vi "Conus_USB.vi"() -> ()   [LabVIEW 2017]
doc: "Conus USB - Versió bàsica de Conus / Sols adquisició i informe"
uses:
  Instance           2 17Saved   Conus_USB .vi
  Instance           1 17Saved   Conus_USB .vi
  Instance           4 17Saved   Conus_USB .vi
  <vilib>/DAQmx/read.llb/DAQmx Read (Digital 1D Bool NChan 1Samp 1Line).vi
  <vilib>/DAQmx/write.llb/DAQmx Write (Digital 1D Bool NChan 1Samp 1Line).vi
  Control 1.ctl
panel:
  in  "ResetExten":bool caption="TARA"
  in  "Bt_Ini_Exten":bool caption="TARA"
  out "CarregaConfig":bool caption="First time"
  out "IndexCel":u8
  out "Mante_a_Vel_0":bool
  out "Fent_Rep":bool
  out "Booleans":refnum<vi>[](array[refnum])
  in  "Rep. Fetes":u8 caption="N. Rep."
  in  "Salir":bool
  in  "EtiquetaTipusParo":string caption="String"
  in  "Etiqueta Velocitats":string caption="String"
  out "appended array":refnum<vi>[](array[refnum])
  out "MissatgesUsuari":string[](array[string])
  out "Caselles":refnum<vi>[](array[refnum])
  out "StringsEstatMáquina":string[](array[string])
  in  "Rep. A Fer":sgl caption="N. Rep." format="%#_1g"
  out "ParoDefor":bool caption="ParoRotura"
  out "ParoDeforFet":bool caption="ParoProcessat"
  out "ParoCargaFet":bool caption="ParoProcessat"
  out "ParoCarga":bool caption="ParoProcessat"
  in  "CaptadorD":u16(ring) caption="Unidades" items=["Deformación", "Extensómetro"]
  in  "FinalEnsayo":bool caption="Final ensayo"
  in  "ActivaParoCarga":bool caption="ActivaParoDefor"
  in  "ValorParoCarga":sgl caption="Fuerza" min=0 format="%#.3f"
  in  "ActivaParoDefor":bool
  in  "ActivaParoRotura":T1
  in  "ValorParoDesplazamiento":sgl caption="Deformación" min=0 format="%#.3f"
  in  "ValorParoRotura":sgl caption="Rotura (%)" min=0 format="%#_3f"
  out "Ensayo activo":bool caption="Prueba en curso"
  out "ArraiMostresxProva":dbl[](array[numeric])
  out "NMostres":dbl
  in  "BtEliminarUltima":bool=TRUE caption="Eliminar última prueba"
  out "Estado ensayo:":string
  out "CodiAturada":u32
  out "ViuMotor":bool
  out "MotorBipolar":bool
  out "Baixar":bool
  out "Pujar":bool
  out "PrimerCaptador":i32
  out "rings":refnum<vi>[](array[refnum])
  in  "IndexUnitatsD":u8
  in  "IndexUnitatsF":u8
  in  "IndexCaptadorD":u8
  in  "IndexCaptadorF":u8
  out "EtiquetesRegistre":string[](array[string])
  out "start":bool
  out "Active_motor":bool
  in  "Inici x Boto":bool
  out "ExtenPoten":bool caption="Extensòmetre Pot."
  out "ValorSenseTara":dbl
  in  "VelocitatMàxima":dbl
  in  "PerCentPrecarga":sgl=0.5 caption="Precarga (%)"
  in  "Precarga":bool
  in  "BtMaxF":bool
  in  "CaptadorF":u16(ring) caption="Unidades" items=["100 kg"=7, "No presente"=24]
  in  "UnidadesF":u16(ring) caption="Unidades" items=["kg"=0, "N"=1, "daN"=3, "KN"=5]
  in  "BtTaraF":bool caption="TARA"
  out "Fuerza":sgl format="%.2f"
  out "Nº Tests":u8 caption="Tests:"
  out "Sobrecarga":bool
  out "Paro Manual":bool
  out "FCI":bool
  out "FCS":bool
  in  "ResoExten":i8(ring) caption="Resolució Extensometre" items=["0.1", "0.2", "0.5", "0.01", "0.02", "0.05", "0.001", "0.002", "0.005"]
  out "PrecargaOn":bool
  in  "ValorPrecarga":dbl caption="Precarga (%)"
  out "Calibratge D":dbl[](array[numeric])
  out "Extensometre":bool
  in  "UnidadesD":u16(ring) caption="Unidades" items=["mm", "inch"]
  in  "BtTaraD":bool caption="TARA"
  out "Deformacion":sgl caption="Deformación" format="%.1f"
  out "Celula_0":u8
  in  "Células":u8(ring) caption="Célula 1" items=["0.5 kg", "1 Kg", "2 Kg", "5 kg", "10 kg", "20 kg", "50 kg", "100 kg", "200 kg", "300 kg", "500 kg", "1000 kg", "2000 kg", "5000 kg", "10000 kg", "20000 kg", "30000 kg", "P-20 kg", "P-200 kg", "P-500 kg", "P-5000 kg", "P-20000 kg", "P-50 bar", "50000 kg", "No presente"]
  in  "UnidadesF_C2":u16(ring) caption="Unidades" items=["kg"=0, "N"=1, "daN"=3]
  in  "UnidadesF_C1":u16(ring) caption="Unidades" items=["kg"=0, "N"=1, "daN"=3, "KN"=5]
  out "ArraiUnitats":cluster{"String":string, "Value":u16}[](array[cluster])=[{"String"="kg", "Value"=0}, {"String"="N", "Value"=1}, {"String"="g", "Value"=2}, {"String"="daN", "Value"=3}, {"String"="cN", "Value"=4}, {"String"="KN", "Value"=5}, {"String"="lb", "Value"=6}]
  in  "UnitatsF":u8[](array[numeric])
  in  "Velocidad Retorno":sgl caption="Retorno" min=0 max=500 step=1 format="%#.1f"
  in  "Velocidad Ensayo":sgl caption="Ensayo" min=0 max=500 step=1
  out "ValorSobrecargaC2":dbl
  out "Valor de control sobrecarga":dbl
  out "Calibratge":dbl[](array[numeric])
  in  "ParaAssaig":bool
  out "ParoProcessat":bool
  out "Salidas_mando":T2={"HI_down"=TRUE, " LO_down"=TRUE, "HI_up"=TRUE, "*"=TRUE, " LO_up"=TRUE, " start"=TRUE, " Ensayo_down"=TRUE, " Ensayo_up"=TRUE}
  out "VelocitatMotor":dbl min=0.0 max=500.0 step=1.0
  out "TempsLectura":u32=150
  out "Maxim":sgl
  in  "Inhibicio":bool
  in  "Ensayonuevo":bool caption="Ensayo Nuevo"
  in  "Guardar":bool caption="Informe"
  in  "Iniciar / Finalizar":bool=TRUE caption="Finalizar prueba"
  out "TablaFinal":dbl[][](array[numeric])
  out "Tabla":dbl[][](array[numeric])
  in  "Columna":i32
  out "Paro Emergencia":bool
  out "ParoRotura":bool
  out "AssaigMM":bool
  out "DSenseTara":sgl caption="Fuerza - N"
  out "FactorsUnitatsPendents_D":dbl[](array[numeric])
  out "ConversioUnitatsD":dbl[](array[numeric])=[1.0, 9.8756, 1000.0, 0.98]
  in  "DadesAdquirides":dbl[](array[numeric]) format="%#_8g"
  out "FactorsUnitatsPendents_F":dbl[](array[numeric])
  in  "LedAssaig":bool
  out "BaixarMM":bool
  out "PujarMM":bool
  in  "TaraD":sgl
  in  "ValMax":bool
  out "FSenseTara":sgl caption="Fuerza - N"
  in  "TaraF":sgl
  out "Password":string
  out "ValorSobrecargaC1":dbl
  out "ConversioUnitatsF":dbl[](array[numeric])=[1.0, 9.8756, 2.2]
  out "Pendents":dbl[](array[numeric]) format="%#_8g"
  in  "Procesa datos":bool
  in  "Stop":bool=TRUE
  in  "First time":bool
  out "?":cluster{"Y":dbl[], "Y":dbl[]}[](graph)
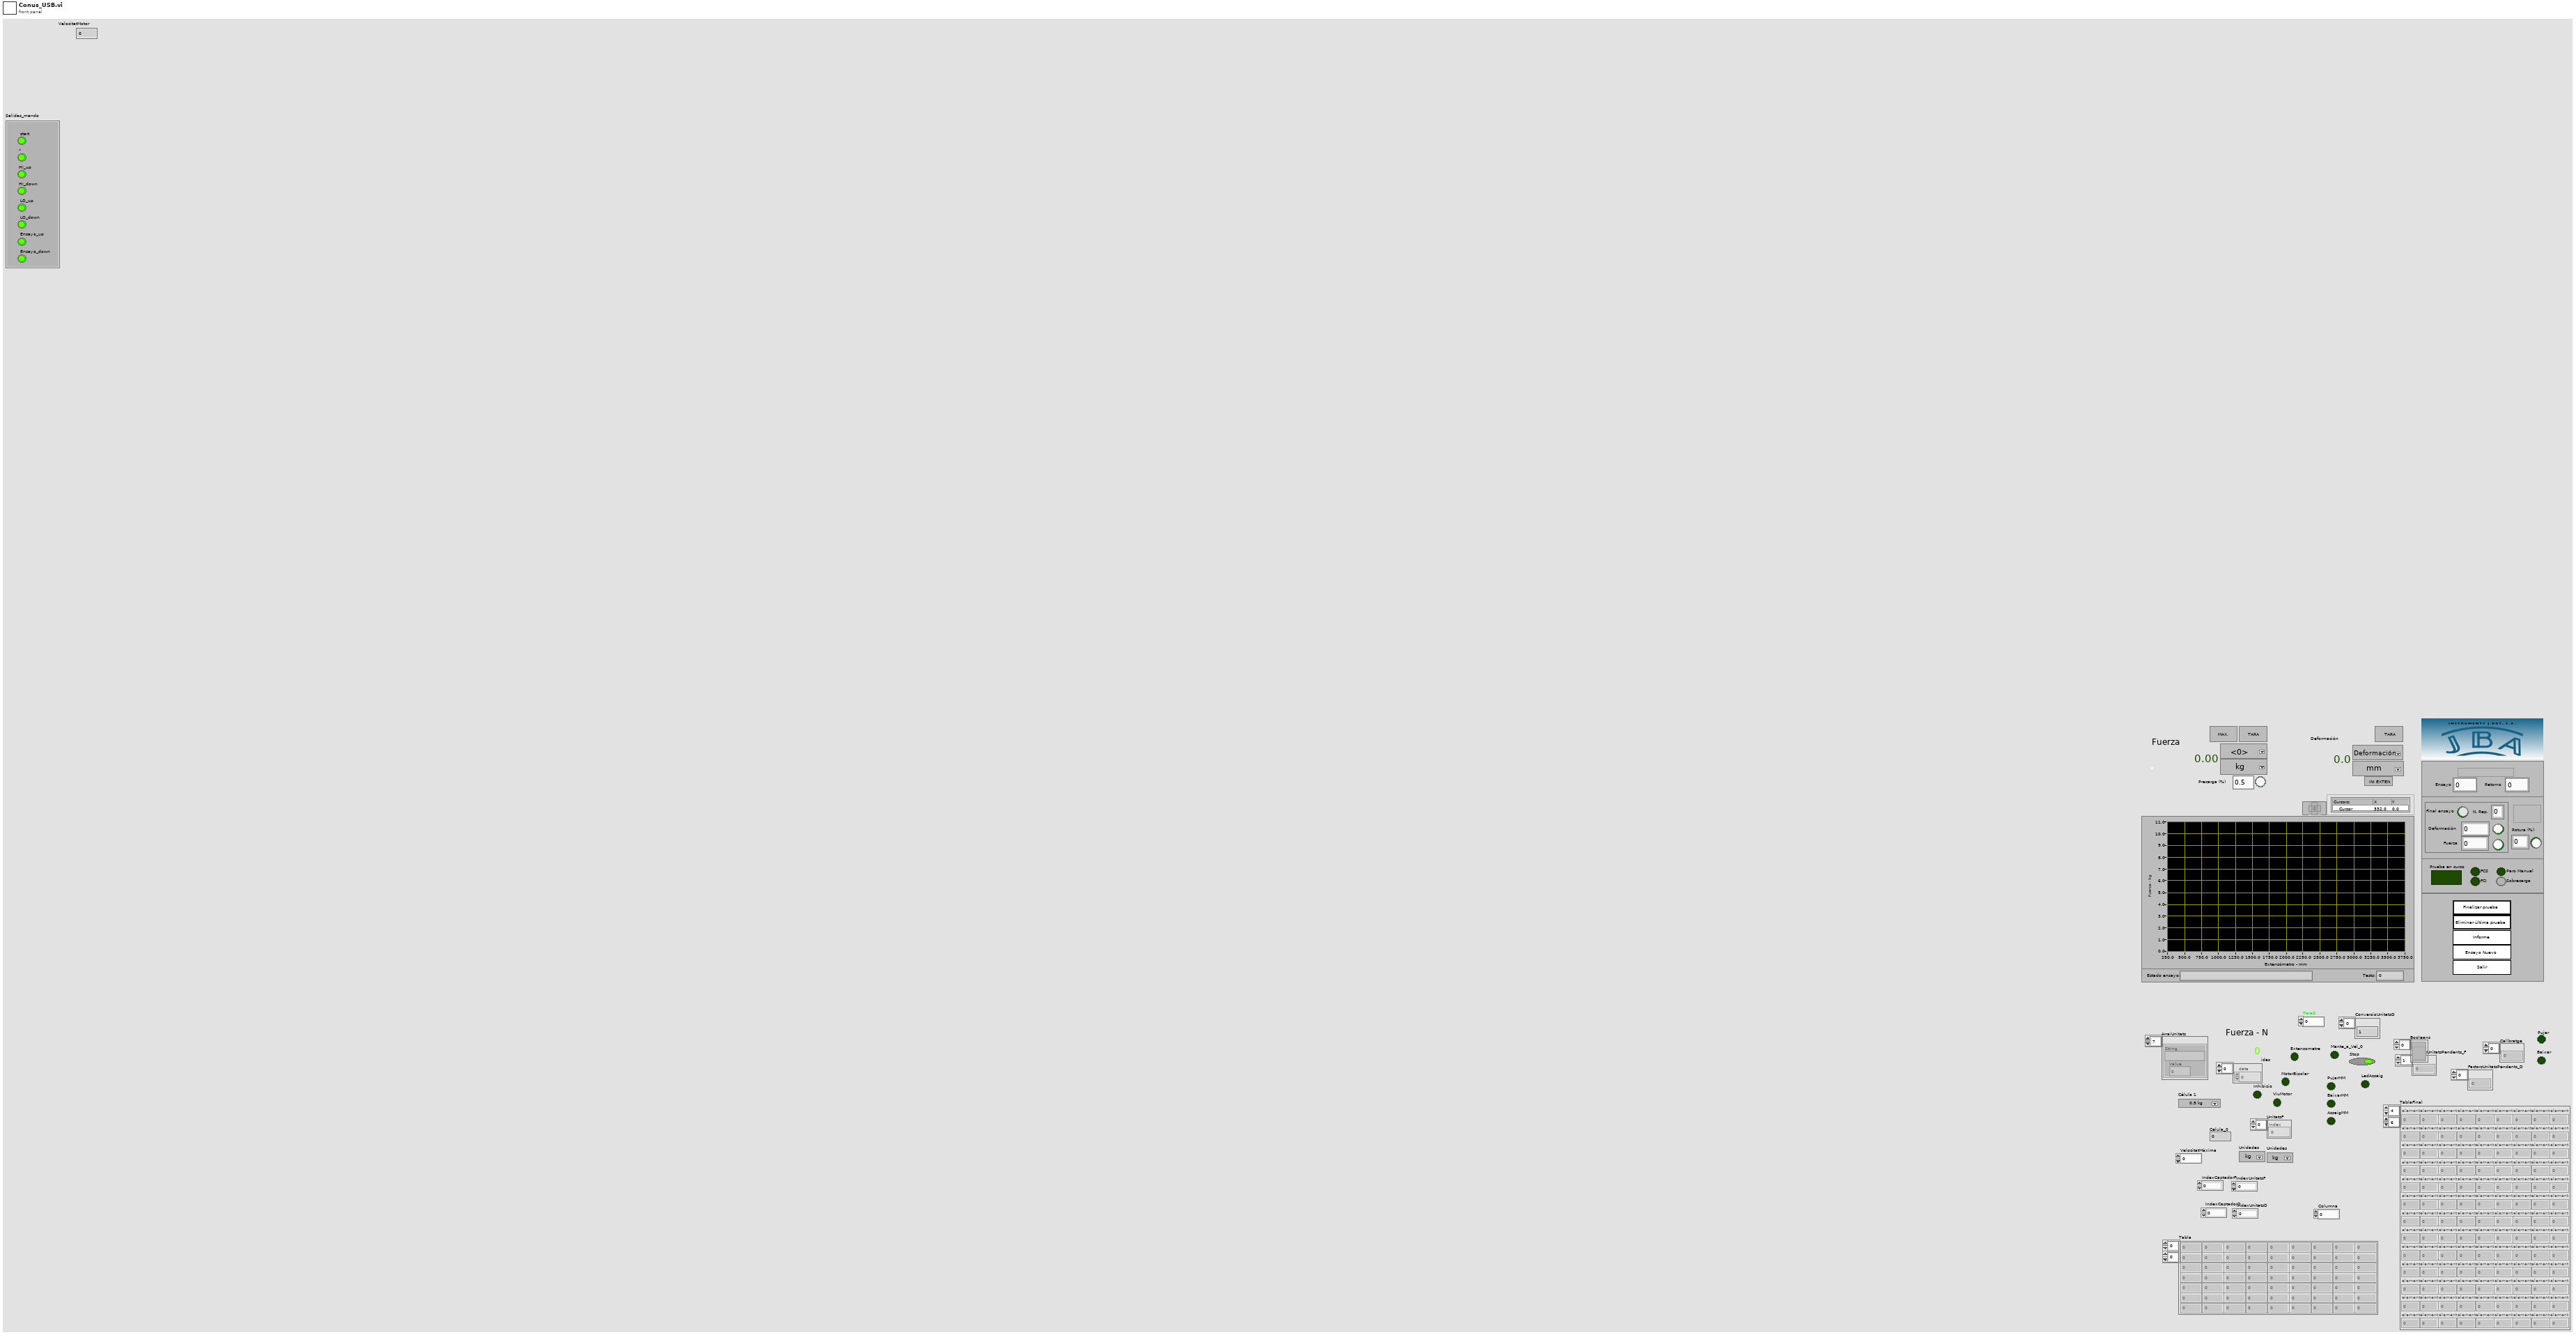
[diagram p1: front panel]
types:
  T1 = typedef "Control 1.ctl" = bool
  T2 = cluster{"HI_down":bool, " LO_down":bool, "HI_up":bool, "*":bool, " LO_up":bool, " start":bool, " Ensayo_down":bool, " Ensayo_up":bool}
  T3 = cluster{"HI_down":bool, "LO_down":bool, "HI_up":bool, "*":bool, "LO_up":bool, "start":bool, "Ensayo_down":bool, "Ensayo_up":bool}
  T4 = typedef "LVStringsAndValuesArrayTypeDef_U8.ctl" = cluster{"String":string, "Value":u8}[]
  T5 = cluster{"Boolean":bool, "element":bool, "Boolean":bool, "Boolean":bool}
  T6 = enum16{"Left Button", "Center Button", "Right Button", "Window Close"}
  T7 = typedef "LVStringsAndValuesArrayTypeDef_U16.ctl" = cluster{"String":string, "Value":u16}[]
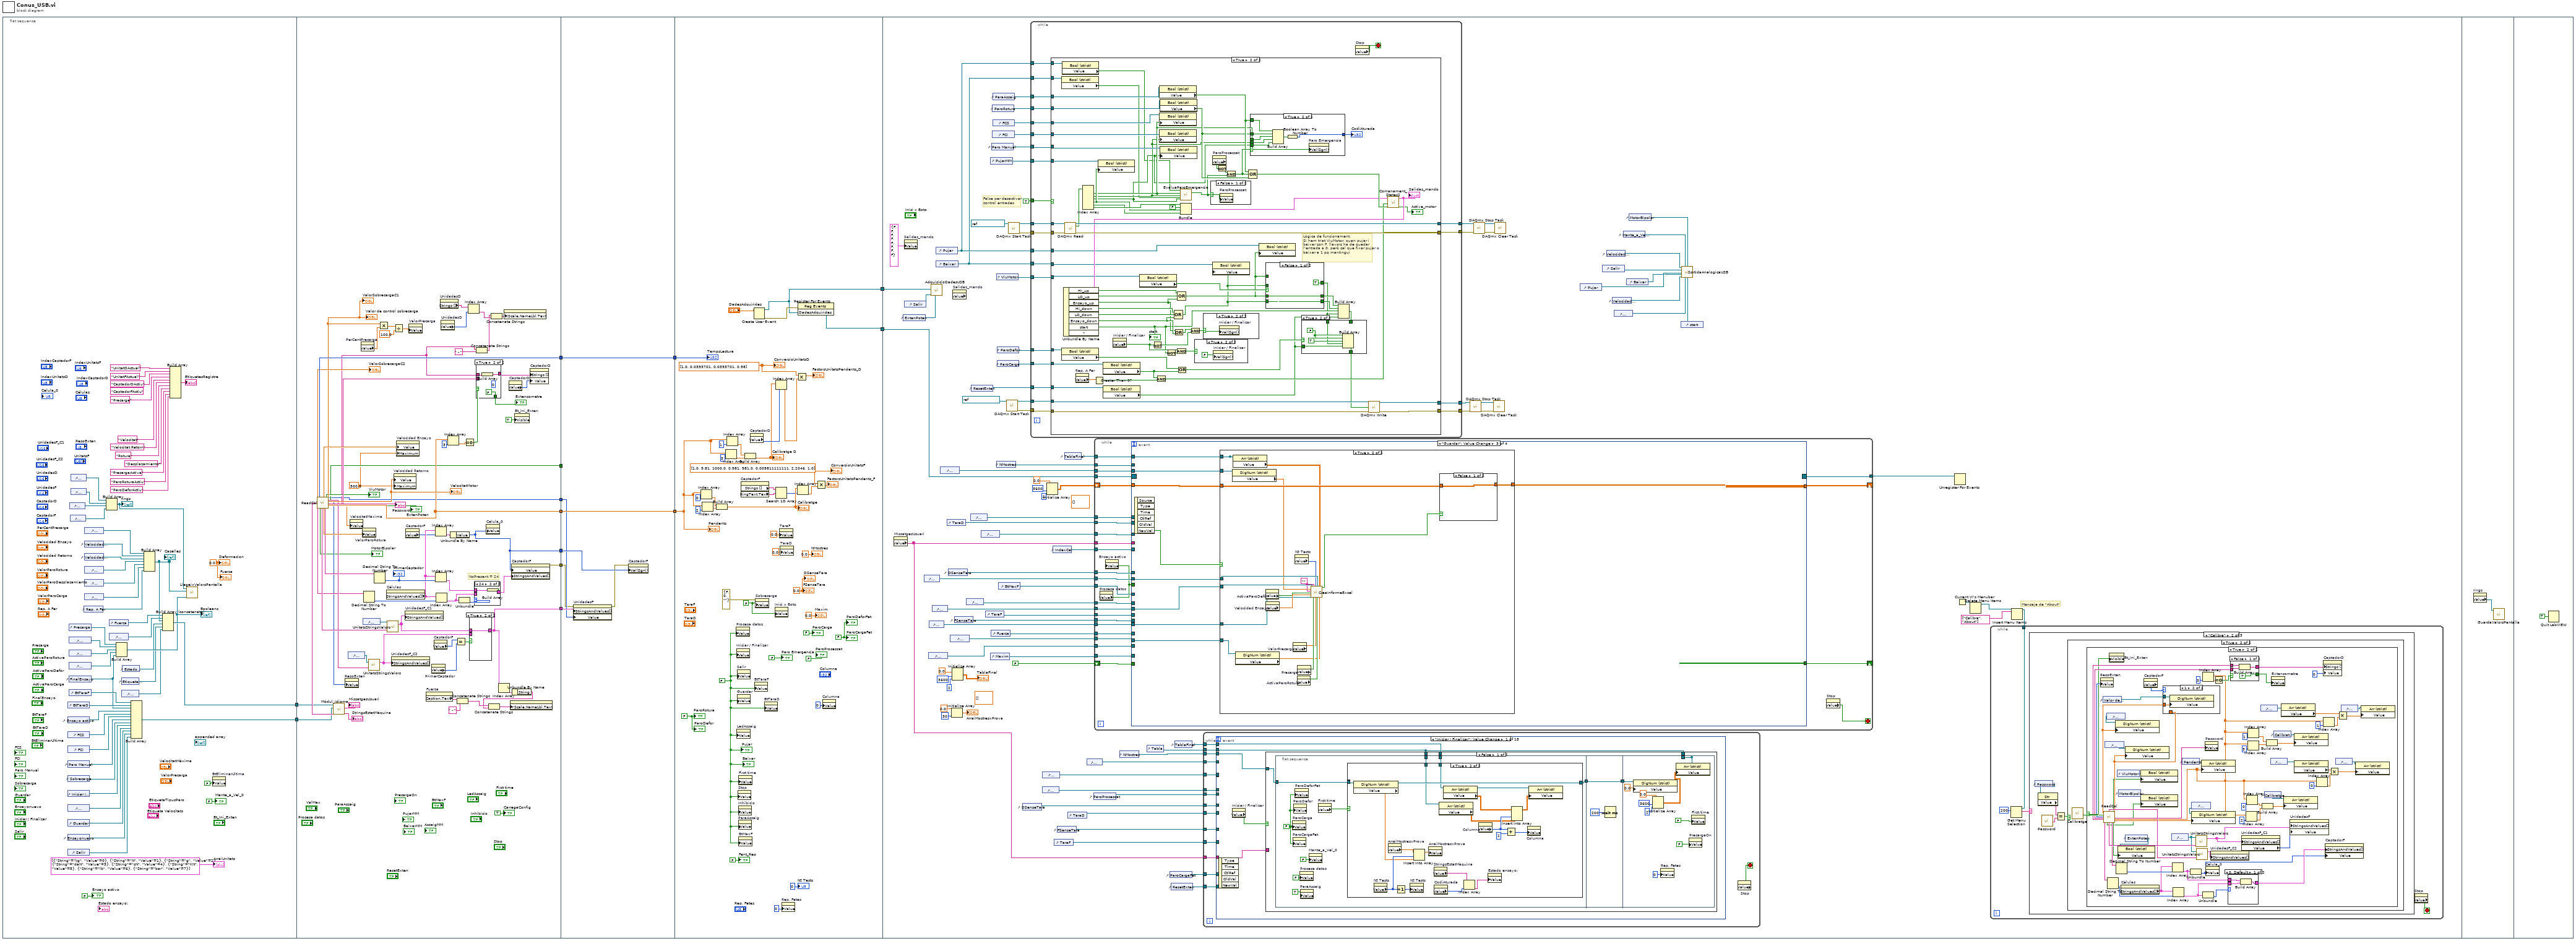
[diagram p0: block diagram]
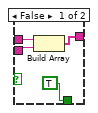
[diagram p3: hidden frame]
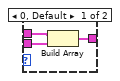
[diagram p4: hidden frame]
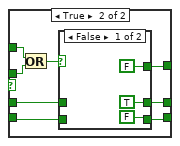
[diagram p7: hidden frame]
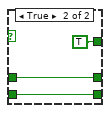
[diagram p8: hidden frame]
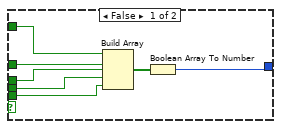
[diagram p11: hidden frame]
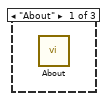
[diagram p13: hidden frame]
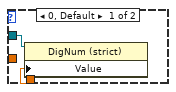
[diagram p16: hidden frame]
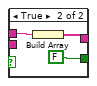
[diagram p17: hidden frame]
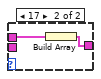
[diagram p18: hidden frame]
diagram:
  n1 = flat-sequence {
    tunnel: [w68] -> w7
    tunnel: [w67] -> w6
    tunnel: [w121] -> w13
    tunnel: [w136] -> w12
    tunnel: w7 -> [w79]
    tunnel: w6 -> [w81]
    tunnel: [w78] -> w5
    tunnel: [w77] -> w4
    tunnel: [w76] -> w3
    tunnel: [w75] -> w2
    tunnel: [w74] -> w1
    tunnel: w13 -> [w159]
    tunnel: [w159] -> w11
    tunnel: w12 -> [w158]
    tunnel: [w158] -> w10
    tunnel: w5 -> [_]
    tunnel: w4 -> [w154]
    tunnel: w3 -> [w157]
    tunnel: w2 -> [w156]
    tunnel: w1 -> [w155]
    tunnel: w11 -> [w178]
    tunnel: [w197] -> w9
    tunnel: [w189] -> w8
    tunnel: w10 -> [w188]
    tunnel: w9 -> [w287]
    tunnel: w8 -> [w270]
    frame #0 {
      w17 = sgl 0.0 ("Deformacion")
      (unwired) "CaptadorFActiu" ("value")
      n2 = control-ref of="BtTaraD"() -> (w42:refnum<vi>)
      n3 = control-ref of="Ensayo activo"() -> (w40:refnum<vi>)
      n4 = control-ref of="FCS"() -> (w39:refnum<vi>)
      n5 = control-ref of="FCI"() -> (w38:refnum<vi>)
      n6 = control-ref of="Paro Manual"() -> (w37:refnum<vi>)
      n7 = control-ref of="Sobrecarga"() -> (w36:refnum<vi>)
      n8 = control-ref of="Iniciar / Finalizar"() -> (w35:refnum<vi>)
      n9 = control-ref of="BtEliminarUltima"() -> (w34:refnum<vi>)
      n10 = control-ref of="Guardar"() -> (w22:refnum<vi>)
      n11 = control-ref of="Ensayonuevo"() -> (w33:refnum<vi>)
      n12 = control-ref of="Salir"() -> (w32:refnum<vi>)
      n13 = control-ref of="Precarga"() -> (w53:refnum<vi>)
      n14 = control-ref of="ActivaParoRotura"() -> (w52:refnum<vi>)
      n15 = control-ref of="ActivaParoDefor"() -> (w51:refnum<vi>)
      n16 = control-ref of="ActivaParoCarga"() -> (w45:refnum<vi>)
      n17 = control-ref of="FinalEnsayo"() -> (w41:refnum<vi>)
      n18 = control-ref of="BtTaraF"() -> (w43:refnum<vi>)
      n19 = control-ref of="CaptadorD"() -> (w48:refnum<vi>)
      n20 = control-ref of="CaptadorF"() -> (w47:refnum<vi>)
      n21 = control-ref of="UnidadesD"() -> (w50:refnum<vi>)
      n22 = control-ref of="UnidadesF"() -> (w49:refnum<vi>)
      n23 = control-ref of="Rep. A Fer"() -> (w15:refnum<vi>)
      n24 = control-ref of="PerCentPrecarga"() -> (w30:refnum<vi>)
      n25 = control-ref of="Velocidad Ensayo"() -> (w29:refnum<vi>)
      n26 = control-ref of="Velocidad Retorno"() -> (w54:refnum<vi>)
      n27 = control-ref of="ValorParoRotura"() -> (w28:refnum<vi>)
      n28 = control-ref of="ValorParoDesplazamiento"() -> (w27:refnum<vi>)
      n29 = control-ref of="ValorParoCarga"() -> (w26:refnum<vi>)
      n30 = Build Array(w50, w49, w48, w47) -> (w46:refnum<vi>[])
      "rings" <- w46
      n31 = control-ref of="Fuerza"() -> (w25:refnum<vi>)
      n32 = control-ref of="Deformacion"() -> (w24:refnum<vi>)
      n33 = Build Array(w53, w52, w51, w45, w41) -> (w31:refnum<vi>[])
      "Booleans" <- w31
      n34 = control-ref of="Etiqueta Velocitats"() -> (w19:refnum<vi>)
      n35 = control-ref of="EtiquetaTipusParo"() -> (w18:refnum<vi>)
      n36 = control-ref of="Estado ensayo:"() -> (w20:refnum<vi>)
      n37 = Build Array(w43, w42, w41, w40, w39, w38, w37, w36, w35, w34, w22, w33, w32) -> (w68:refnum<vi>[])
      n38 = Build Array(w30, w29, w54, w28, w27, w26, w15) -> (w21:refnum<vi>[])
      "Caselles" <- w21
      n39 = Build Array (concatenate)(w25, w24, w21, w20, w19, w18) -> (w67:refnum<vi>[])
      n40 = Build Array("UnitatDActual" ("value"), "UnitatFActual" ("value"), "CaptadorDActiu" ("value"), "Precarga" ("value"), "Velocitat" ("value"), "Velocitat Retorn" ("value"), "Rotura" ("value"), "Desplazamiento" ("value"), "PrecargaActiva" ("value"), "ParoRoturaActiu" ("value"), "ParoDeforActiu" ("value")) -> (→"EtiquetesRegistre":string[])
      n41 = call "LlegeixValorsPantalla.vi"("rings"=w46, "Caselles 2"=w21, "Booleans"=w31) -> ()  [unwired: 8 in]
      n42 = property on="BtEliminarUltima" class="Bool (strict)"("Value"=FALSE ("BtEliminarUltima")) -> ()  [unwired: 2 in, 2 out]
      "Ensayo activo" <- FALSE ("Ensayo activo")
      "Fuerza" <- w17
      "Deformacion" <- w17
      "ArraiUnitats" <- cluster{"String":string, "Value":u16}[] [{"String"="kg", "Value"=0}, {"String"="N", "Value"=1}, {"String"="g", "Value"=2}, {"String"="daN", "Value"=3}, {"String"="cN", "Value"=4}, {"String"="KN", "Value"=5}, {"String"="lb", "Value"=6}, {"String"="bar", "Value"=7}] ("Strings And Values [] 2")
      "Mante_a_Vel_0" <- FALSE ("Mante_a_Vel_0")
    }
    frame #1 {
      w71 = 500.0 ("Data Entry Limits:Maximum")
      # "NoPresent = 24"
      n43 = call "ReadCal.vi"() -> ("SobrecargaC2"=→"ValorSobrecargaC2":dbl, "ResoExten"=w114:i8, "TextExtensometre"=w118:string, "TextDeformacio"=w80:string, "SegonCaptador"=w128:string, "TempsLectura"=w136:u16, "Idioma"=w83:string, "MotorBipolar"=→"MotorBipolar":bool, "UnitatsC2"=w129:string, "UnitatsC1"=w130:string, "Velocitat"=w137:dbl, "ParoRotura"=w138:dbl, "V. Retorn"=w133:dbl, "PrimerCaptador"=w126:string, "ViuMotor"=→"ViuMotor":bool, "ExtenPoten"=→"ExtenPoten":bool, "Unidades"=w74:u8, "Sec?"=w78:bool, "SobrecargaC1"=w115:dbl, "Password"=→"Password":string, "Pendents"=w121:dbl[], "VelocitatMàxima"=w70:dbl)  [unwired: 2 in, 4 out]
      "VelocitatMotor" <- w133
      "ValorSobrecargaC1" <- w115
      "Valor de control sobrecarga" <- w115
      n44 = call "Módul_Idioma.vi"("Idioma"=w83, "Array"=w79, "Caselles"=w81) -> ("TextosEstatMaquina"=→"StringsEstatMáquina":string[], "MissatgesUsuari"=→"MissatgesUsuari":string[])  [unwired: 7 in]
      n45 = property on="ResoExten" class="Ring (strict)"("Value"=w114) -> ()  [unwired: 2 in, 2 out]
      n46 = control-ref of="ArraiUnitats"() -> (w131:refnum<vi>)
      n47 = property on="VelocitatMàxima" class="DigNum (strict)"("Value"=w70) -> ()  [unwired: 2 in, 2 out]
      n48 = property on="PerCentPrecarga" class="DigNum (strict)"() -> ("Value"=w106:sgl)  [unwired: 2 in, 2 out]
      n49 = property on="ValorParoRotura" class="DigNum (strict)"("Value"=w138) -> ()  [unwired: 2 in, 2 out]
      n50 = control-ref of="ArraiUnitats"() -> (w132:refnum<vi>)
      n51 = Decimal String To Number(string=w128) -> (number=w127:i32)  [unwired: 2 in, 1 out]
      n52 = call "UnitatsStringsValors.vi"("UnitatsC1"=w129, "Arr Refnum"=w131) -> ("Array 2"=w96:cluster{"String":string, "Value":u16}[])  [unwired: 1 out]
      n53 = Decimal String To Number(string=w126) -> (number=w125:i32)  [unwired: 2 in, 1 out]
      "PrimerCaptador" <- w125
      n54 = Multiply(x=w115, y=w106) -> (x*y=w117:dbl)
      n55 = property on="Células" class="Ring (strict)"() -> ("StringsAndValues[]"=w103:T4)  [unwired: 2 in, 2 out]
      n56 = call "UnitatsStringsValors.vi"("UnitatsC1"=w130, "Arr Refnum"=w132) -> ("Array 2"=w97:cluster{"String":string, "Value":u16}[])  [unwired: 1 out]
      n57 = property on="UnidadesF_C2" class="Ring (strict)"("StringsAndValues[]"=w96) -> ()  [unwired: 2 in, 2 out]
      n58 = Divide(x=w117, y=100.0) -> (x/y=w112:dbl)
      n59 = property on="Velocidad Retorno" class="DigNum (strict)"("Value"=w133, "Maximum"=w71) -> ()  [unwired: 2 in, 2 out]
      n60 = property on="Velocidad Ensayo" class="DigNum (strict)"("Value"=w137, "Maximum"=w71) -> ()  [unwired: 2 in, 2 out]
      n61 = property on="UnidadesF_C1" class="Ring (strict)"("StringsAndValues[]"=w97) -> ()  [unwired: 2 in, 2 out]
      n62 = property on="CaptadorF" class="Ring (strict)"() -> ("Value"=w101:u16)  [unwired: 2 in, 2 out]
      n63 = property on="ValorPrecarga" class="DigNum (strict)"("Value"=w112) -> ()  [unwired: 2 in, 2 out]
      n64 = property on="Fuerza" class="DigNum (strict)"() -> ("Caption.Text"=w109:string)  [unwired: 2 in, 2 out]
      n65 = property on="PrimerCaptador" class="DigNum (strict)"() -> ("Value"=w98:i32)  [unwired: 2 in, 2 out]
      n66 = property on="CaptadorF" class="Ring (strict)"() -> ("Value"=w99:u16)  [unwired: 2 in, 2 out]
      n67 = Index Array(array=w103, index=w101) -> (element=w102:cluster{"String":string, "Value":u8})
      n68 = Index Array(array=w103, index=w125) -> (element=w105:cluster{"String":string, "Value":u8})
      n69 = Index Array(array=w103, index=w127) -> (element=w123:cluster{"String":string, "Value":u8})
      n70 = property on="UnidadesD" class="Ring (strict)"() -> ("Strings []"=w91:string[])  [unwired: 2 in, 2 out]
      n71 = property on="UnidadesD" class="Ring (strict)"() -> ("Value"=w90:u16)  [unwired: 2 in, 2 out]
      n72 = Index Array(array=w121, index=3) -> (element=w119:dbl)
      n73 = Unbundle By Name(w102) -> ("Value"=w76:u8)
      n74 = Equal?(x=w99, y=w98) -> (x = y?=w100:bool)
      n75 = Concatenate Strings(w109, " - ") -> (w108:string)
      n76 = Unbundle(w123) -> ("Value"=w124:u8)  [unwired: 1 out]
      n77 = Equal To 0?(x=w119) -> (x = 0?=w122:bool)
      n78 = Index Array(array=w91, index=w90) -> (element=w89:string)
      n79 = case shown="True" w100 {
        tunnel: w97 -> [_ w140]
        tunnel: [w139 w140] -> w75
        tunnel: w96 -> [w139 _]
        frame False {
        }
        frame True {
        }
      }
      n80 = case shown="24" w124 {
        tunnel: w105 -> [w150 w151]
        tunnel: w123 -> [w149 _]
        tunnel: [w148 w152] -> w104
        frame 0, Default {
          n81 = Build Array(w150, w149) -> (w148:cluster{"String":string, "Value":u8}[])
        }
        frame 24 {
          n82 = Build Array(w151) -> (w152:cluster{"String":string, "Value":u8}[])
        }
      }
      n83 = Concatenate Strings(w80, " - ") -> (w87:string)
      n84 = case shown="True" w122 {
        tunnel: w118 -> [w144 _]
        tunnel: [w143 w145] -> w92
        tunnel: [TRUE ("Extensometre") FALSE ("Extensometre")] -> w72
        tunnel: w80 -> [w141 w146]
        frame False {
          n85 = Build Array(w141, w144) -> (w143:string[])
        }
        frame True {
          (unwired) 0 ("index")
          n86 = Build Array(w146) -> (w145:string[])
        }
      }
      "Extensometre" <- w72
      n87 = property on="Celula_0" class="DigNum (strict)"("Value"=w76) -> ()  [unwired: 2 in, 2 out]
      n88 = Concatenate Strings(w87, w89) -> (w107:string)
      n89 = Index Array(array=w75) -> (element=w94:cluster{"String":string, "Value":u16})  [unwired: 1 in]
      n90 = property class="XYGraph (strict)"("XScale.NameLbl.Text"=w107) -> ()  [unwired: 2 in, 2 out]
      n91 = property on="CaptadorD" class="Ring (strict)"() -> ("Value"=w93:u16)  [unwired: 2 in, 2 out]
      n92 = property on="CaptadorF" class="Ring (strict)"("Value"=w76, "StringsAndValues[]"=w104) -> (error out=w77:errorcluster)  [unwired: 2 in, 1 out]
      n93 = Unbundle By Name(w94) -> ("String"=w95:string)
      n94 = Concatenate Strings(w108, w95) -> (w113:string)
      n95 = property class="XYGraph (strict)"("YScale.NameLbl.Text"=w113) -> ()  [unwired: 2 in, 2 out]
      n96 = property on="Bt_Ini_Exten" class="Bool (strict)"("Visible"=TRUE) -> ()  [unwired: 2 in, 2 out]
      n97 = property on="CaptadorD" class="Ring (strict)"("Strings []"=w92, "Value"=w93) -> ()  [unwired: 2 in, 2 out]
      "CarregaConfig" <- TRUE ("CarregaConfig")
    }
    frame #2 {
      n98 = property on="UnidadesF" class="Ring (strict)"(error in=w154, "StringsAndValues[]"=w156, "Value"=w155) -> (error out=w153:errorcluster)  [unwired: 1 in, 1 out]
      n99 = property on="CaptadorF" class="Ring (strict)"(error in=w153, "Val(Sgnl)"=w157) -> ()  [unwired: 1 in, 2 out]
    }
    frame #3 {
      w163 = FALSE ("ParoCargaFet")
      w162 = FALSE ("ParoRotura")
      w176 = dbl[] [1.0, 0.0393701, 0.0393701, 0.98]
      w191 = sgl 0.0 ("FSenseTara")
      w199 = dbl[] [1.0, 9.81, 1000.0, 0.981, 981.0, 0.009811111111, 2.2046, 1.0]
      w170 = FALSE ("Sobrecarga")
      w166 = FALSE ("Iniciar / Finalizar")
      n100 = Index Array(array=w178, index=0) -> (element=w184:dbl)
      n101 = Index Array(array=w178, index=2) -> (element=w185:dbl)
      n102 = Build Array(w184, w185) -> (w183:dbl[])
      "Calibratge" <- w183
      n103 = Index Array(array=w178, index=3) -> (element=w179:dbl)
      n104 = Index Array(array=w178, index=1) -> (element=w177:dbl)
      n105 = property on="Procesa datos" class="Bool (strict)"("Value"=w166) -> ()  [unwired: 2 in, 2 out]
      n106 = property on="Iniciar / Finalizar" class="Bool (strict)"("Value"=w166) -> ()  [unwired: 2 in, 2 out]
      n107 = property on="LedAssaig" class="Bool (strict)"("Value"=w166) -> ()  [unwired: 2 in, 2 out]
      n108 = property on="Salir" class="Bool (strict)"("Value"=w166) -> ()  [unwired: 2 in, 2 out]
      n109 = property on="Guardar" class="Bool (strict)"("Value"=w166) -> ()  [unwired: 2 in, 2 out]
      n110 = property on="Stop" class="Bool (strict)"("Value"=w166) -> ()  [unwired: 2 in, 2 out]
      n111 = property on="Inhibicio" class="Bool (strict)"("Value"=w166) -> ()  [unwired: 2 in, 2 out]
      n112 = property on="ParaAssaig" class="Bool (strict)"("Value"=w166) -> ()  [unwired: 2 in, 2 out]
      n113 = property on="First time" class="Bool (strict)"("Value"=w166) -> ()  [unwired: 2 in, 2 out]
      n114 = property on="BtMaxF" class="Bool (strict)"("Value"=w166) -> ()  [unwired: 2 in, 2 out]
      n115 = property on="CaptadorF" class="Ring (strict)"() -> ("Strings []"=w169:string[], "RingText.Text"=w168:string)  [unwired: 2 in, 2 out]
      n116 = Build Array(w177, w179) -> (w174:dbl[])
      "Calibratge D" <- w174
      n117 = property on="CaptadorD" class="Ring (strict)"() -> ("Value"=w175:u16)  [unwired: 2 in, 2 out]
      n118 = Create User Event(user event datatype="DadesAdquirides") -> (user event=w189:refnum<user-event>, error out=w196:errorcluster)  [unwired: 1 in]
      n119 = property on="BtTaraF" class="Bool (strict)"("Value"=w166) -> ()  [unwired: 2 in, 2 out]
      n120 = property on="Sobrecarga" class="Bool (strict)"(error in=errorcluster {"status"=FALSE, "code"=0, "source"=""} ("error in (no error)"), "Value"=w170) -> ()  [unwired: 1 in, 2 out]
      n121 = property on="BtTaraD" class="Bool (strict)"("Value"=w166) -> ()  [unwired: 2 in, 2 out]
      n122 = property on="Inici x Boto" class="Bool (strict)"("Value"=w170) -> ()  [unwired: 2 in, 2 out]
      n123 = Index Array(array=w174, index=w175) -> (element=w173:dbl)
      n124 = Search 1D Array(1D array=w169, element=w168) -> (index of element=w167:i32)  [unwired: 1 in]
      n125 = property on="TaraF" class="DigNum (strict)"("Value"=sgl 0.0 ("Tara")) -> ()  [unwired: 2 in, 2 out]
      n126 = property on="TaraD" class="DigNum (strict)"("Value"=sgl 0.0 ("TaraD")) -> ()  [unwired: 2 in, 2 out]
      n127 = property on="Rep. Fetes" class="DigNum (strict)"("Value"=u8 0 ("Rep. Fetes")) -> ()  [unwired: 2 in, 2 out]
      n128 = Multiply(x=w176, y=w173) -> (x*y=→"FactorsUnitatsPendents_D":dbl[])
      n129 = Index Array(array=w183, index=w167) -> (element=w182:dbl)
      n130 = register-events(error in=w196, w189) -> (reference out=w197:refnum<event-registration>)  [unwired: 1 in, 1 out]
      n131 = Multiply(x=w199, y=w182) -> (x*y=→"FactorsUnitatsPendents_F":dbl[])
      n132 = property on="Columna" class="DigNum (strict)"("Value"=0 ("Columna")) -> ()  [unwired: 2 in, 2 out]
      "Pendents" <- w178
      "ConversioUnitatsF" <- w199
      "FSenseTara" <- w191
      "ConversioUnitatsD" <- w176
      "DSenseTara" <- w191
      "ParoRotura" <- w162
      "Paro Emergencia" <- FALSE ("Paro Emergencia")
      "Maxim" <- sgl 0.0 ("Maxim")
      "TempsLectura" <- w188
      "ParoProcessat" <- FALSE ("ParoProcessat")
      "Nº Tests" <- u8 0 ("Nº Tests")
      "Pujar" <- w166
      "Baixar" <- w166
      "NMostres" <- 0.0 ("NMostres")
      "ParoCarga" <- FALSE ("ValorCargaFet")
      "ParoCargaFet" <- w163
      "ParoDeforFet" <- w163
      "ParoDefor" <- w162
      "Fent_Rep" <- FALSE ("Fent_Rep")
    }
    frame #4 {
      (unwired) dbl[][] []
      (unwired) dbl[][] [] ("TablaFinal")
      # "False per desactivar\ncontrol entrades"
      # "Mensaje de \"About\""
      n133 = property on="MissatgesUsuari" class="Arr (strict)"() -> ("Value"=w217:string[])  [unwired: 2 in, 2 out]
      n134 = control-ref of="ExtenPoten"() -> (w237:refnum<vi>)
      n135 = property on="Salidas_mando" class="Clust (strict)"("Value"=T3 {"HI_down"=FALSE, "LO_down"=FALSE, "HI_up"=FALSE, "*"=FALSE, "LO_up"=FALSE, "start"=FALSE, "Ensayo_down"=FALSE, "Ensayo_up"=FALSE} ("Salidas_mando")) -> ()  [unwired: 2 in, 2 out]
      n136 = control-ref of="Salir"() -> (w271:refnum<vi>)
      n137 = control-ref of="UnidadesD"() -> (w280:refnum<vi>)
      n138 = control-ref of="ValorParoCarga"() -> (w222:refnum<vi>)
      n139 = control-ref of="CaptadorF"() -> (w246:refnum<vi>)
      n140 = call "AdquisicioDadesUSB.vi"("ExtensometrePoten"=w237, "Stop"=w271, "user event"=w270) -> ()  [unwired: 9 in]
      n141 = control-ref of="UnidadesF"() -> (w279:refnum<vi>)
      n142 = control-ref of="Pujar"() -> (w228:refnum<vi>)
      n143 = control-ref of="Baixar"() -> (w227:refnum<vi>)
      n144 = control-ref of="ValorParoDesplazamiento"() -> (w242:refnum<vi>)
      n145 = control-ref of="TaraD"() -> (w283:refnum<vi>)
      n146 = control-ref of="DSenseTara"() -> (w284:refnum<vi>)
      n147 = control-ref of="ValorParoRotura"() -> (w276:refnum<vi>)
      n148 = Initialize Array(0.0 ("element"), 30 ("dimension size")) -> (→"ArraiMostresxProva":dbl[])
      n149 = Initialize Array(0.0 ("element"), 3600 ("dimension size"), 2 ("dimension size")) -> (→"TablaFinal":dbl[][])
      n150 = property on="Salidas_mando" class="Clust (strict)" props=["Value"]() -> ()  [unwired: 2 in, 3 out]
      n151 = control-ref of="FSenseTara"() -> (w289:refnum<vi>)
      n152 = control-ref of="FactorsUnitatsPendents_F"() -> (w288:refnum<vi>)
      n153 = control-ref of="FactorsUnitatsPendents_D"() -> (w286:refnum<vi>)
      n154 = control-ref of="ResetExten"() -> (w209:refnum<vi>)
      n155 = control-ref of="Deformacion"() -> (w285:refnum<vi>)
      n156 = control-ref of="TaraF"() -> (w290:refnum<vi>)
      n157 = control-ref of="PujarMM"() -> (w230:refnum<vi>)
      n158 = control-ref of="Maxim"() -> (w269:refnum<vi>)
      n159 = control-ref of="Fuerza"() -> (w239:refnum<vi>)
      n160 = control-ref of="Paro Manual"() -> (w250:refnum<vi>)
      n161 = control-ref of="ParoRotura"() -> (w249:refnum<vi>)
      n162 = control-ref of="FCI"() -> (w251:refnum<vi>)
      n163 = control-ref of="ParaAssaig"() -> (w248:refnum<vi>)
      n164 = control-ref of="FCS"() -> (w252:refnum<vi>)
      n165 = control-ref of="ViuMotor"() -> (w231:refnum<vi>)
      n166 = control-ref of="NMostres"() -> (w223:refnum<vi>)
      n167 = control-ref of="ParoDefor"() -> (w220:refnum<vi>)
      n168 = control-ref of="ParoCarga"() -> (w221:refnum<vi>)
      n169 = control-ref of="BtMaxF"() -> (w244:refnum<vi>)
      n170 = call <vilib>:"DAQmx Start Task.vi"("task/channels in"=refnum<k21> "USBDigitalOut") -> ("task out"=w258:refnum<k21>, "error out"=w257:errorcluster)  [unwired: 13 in]
      n171 = call <vilib>:"DAQmx Start Task.vi"("task/channels in"=refnum<k21> "USBDigitalIn") -> ("task out"=w266:refnum<k21>, "error out"=w265:errorcluster)  [unwired: 13 in]
      n172 = control-ref of="DSenseTara"() -> (w281:refnum<vi>)
      n173 = while {
        tunnel: w266 -> [w317]
        tunnel: w265 -> [w316]
        tunnel: [w315] -> w261
        tunnel: [w314] -> w260
        tunnel: w258 -> [w313]
        tunnel: w257 -> [w312]
        tunnel: [w311] -> w254
        tunnel: [w310] -> w253
        tunnel: w252 -> [w309]
        tunnel: w251 -> [w308]
        tunnel: w250 -> [w307]
        tunnel: w249 -> [w306]
        tunnel: w248 -> [w305]
        tunnel: TRUE -> [w304]
        tunnel: w228 -> [w302]
        tunnel: w227 -> [w301]
        tunnel: w231 -> [w300]
        tunnel: w230 -> [w299]
        tunnel: w227 -> [w298]
        tunnel: w228 -> [w297]
        tunnel: w221 -> [w296]
        tunnel: w220 -> [w295]
        tunnel: w209 -> [w294]
        stop <- w303 stop-if-true
        n174 = case shown="True" w304 {
          tunnel: w317 -> [w321 w392]
          tunnel: w316 -> [w320 w391]
          tunnel: [w321 w390] -> w315
          tunnel: [w320 w389] -> w314
          tunnel: w313 -> [w319 w384]
          tunnel: w312 -> [w318 w383]
          tunnel: [w318 w382] -> w311
          tunnel: [w319 w381] -> w310
          tunnel: w309 -> [_ w378]
          tunnel: w308 -> [_ w377]
          tunnel: w307 -> [_ w376]
          tunnel: w306 -> [_ w369]
          tunnel: w305 -> [_ w366]
          tunnel: w302 -> [_ w359]
          tunnel: w301 -> [_ w358]
          tunnel: w300 -> [_ w356]
          tunnel: w299 -> [_ w346]
          tunnel: w298 -> [_ w343]
          tunnel: w297 -> [_ w342]
          tunnel: w296 -> [_ w333]
          tunnel: w295 -> [_ w332]
          tunnel: w294 -> [_ w324]
          frame False {
          }
          frame True {
            # "Lògica de funcionament.\nSi hem triat ViuMotor, quan pujar i baixar son F, llavors ha de quedar l'entrada a 0, però cal que fixar pujar o baixar a 1 pq mantingui"
            n175 = property class="Bool (strict)"(reference=w343) -> ("Value"=w336:bool)  [unwired: 1 in, 2 out]
            n176 = property class="Bool (strict)"(reference=w332) -> ("Value"=w331:bool)  [unwired: 1 in, 2 out]
            n177 = property class="Bool (strict)"(reference=w342) -> ("Value"=w337:bool)  [unwired: 1 in, 2 out]
            n178 = call-poly <vilib>:"DAQmx Read.vi"("task/channels in"=w392, "error in"=w391) -> ("task out"=w390:refnum<k21>, "data"=w350:bool[], "error out"=w389:errorcluster)  [unwired: 11 in]
            n179 = property on="Rep. A Fer" class="DigNum (strict)"() -> ("Value"=w328:sgl)  [unwired: 2 in, 2 out]
            n180 = Index Array(array=w350) -> (element #1=w340:bool, element #2=w339:bool, element #3=w338:bool, element #4=w344:bool, element #5=w345:bool, element #6=w380:bool)  [unwired: 6 in]
            n181 = Greater Than 0?(x=w328) -> (x > 0?=w326:bool)
            n182 = property class="Bool (strict)"(reference=w346, "Value"=w344) -> ()  [unwired: 1 in, 2 out]
            n183 = property class="Bool (strict)"(reference=w333) -> ("Value"=w327:bool)  [unwired: 1 in, 2 out]
            n184 = property class="Bool (strict)"(reference=w324) -> ("Value"=w322:bool)  [unwired: 1 in, 2 out]
            n185 = property on="Iniciar / Finalizar" class="Bool (strict)"() -> ("Value"=w363:bool)  [unwired: 2 in, 2 out]
            n186 = property class="Bool (strict)"(reference=w356) -> ("Value"=w355:bool)  [unwired: 1 in, 2 out]
            n187 = Not(x=w363) -> (.not. x?=w371:bool)
            n188 = And(x=w327, y=w326) -> (x .and. y?=w325:bool)
            n189 = property class="Bool (strict)"(reference=w366) -> ("Value"=w349:bool)  [unwired: 1 in, 2 out]
            n190 = property class="Bool (strict)"(reference=w378, "Value"=w340) -> ()  [unwired: 1 in, 2 out]
            n191 = property class="Bool (strict)"(reference=w377, "Value"=w339) -> ()  [unwired: 1 in, 2 out]
            n192 = property class="Bool (strict)"(reference=w369) -> ("Value"=w348:bool)  [unwired: 1 in, 2 out]
            n193 = property class="Bool (strict)"(reference=w376, "Value"=w338) -> ()  [unwired: 1 in, 2 out]
            n194 = Or(x=w331, y=w327) -> (x .or. y?=w330:bool)
            n195 = Bundle("Boolean"=w380, "element"=FALSE, "Boolean"=w344, "Boolean"=w345) -> (w329:T5)  [unwired: 1 in]
            n196 = call "EvaluaParoEmergencia.vi"("EsticPujant"=w337, "FCI"=w339, "FCS"=w340, "EsticBaixant"=w336, "ParoManual"=w338) -> ("Paro"=w341:bool)  [unwired: 10 in]
            n197 = case shown="False" w341 {
              selector: w341 -> [w417 _]
              frame False {
                n198 = property on="ParoProcessat" class="Bool (strict)"("Value"=w417) -> ()  [unwired: 2 in, 2 out]
              }
              frame True {
              }
            }
            n199 = property on="ParoProcessat" class="Bool (strict)"() -> ("Value"=w368:bool)  [unwired: 2 in, 2 out]
            n200 = Not(x=w368) -> (.not. x?=w367:bool)
            n201 = And(x=w367, y=w341) -> (x .and. y?=w365:bool)
            n202 = Compound Arithmetic op=OR(w349, w365, w348) -> (w364:bool)
            n203 = case shown="True" w365 {
              selector: w365 -> [_ w432]
              tunnel: w349 -> [w423 w431]
              tunnel: w348 -> [w422 w430]
              tunnel: w340 -> [w421 w429]
              tunnel: w339 -> [w420 w428]
              tunnel: w338 -> [w419 w427]
              tunnel: [w418 w425] -> w347
              frame False {
                n204 = Build Array(w423, w422, w421, w420, w419) -> (w424:bool[])
                n205 = Boolean Array To Number(Boolean array=w424) -> (number=w418:u32)
              }
              frame True {
                n206 = Build Array(w431, w430, w429, w428, w427) -> (w426:bool[])
                n207 = Boolean Array To Number(Boolean array=w426) -> (number=w425:u32)
                n208 = property on="Paro Emergencia" class="Bool (strict)"("Val(Sgnl)"=w432) -> ()  [unwired: 2 in, 2 out]
              }
            }
            "CodiAturada" <- w347
            n209 = call "Comanament_States2.vi"("Emergencia"=w364, "ReseUpDown"=w325, "Entradas_Botones"=w329) -> ("Active_motor"=→"Active_motor":bool, "Salidas_mando"=w370:T2)  [unwired: 5 in]
            "Salidas_mando" <- w370
            n210 = Unbundle By Name(w370) -> ("HI_up"=w388:bool, "LO_up"=w387:bool, "Ensayo_up"=w374:bool, "HI_down"=w386:bool, "LO_down"=w385:bool, "Ensayo_down"=w375:bool, "start"=w357:bool)  [unwired: 1 out]
            "start" <- w357
            n211 = Not(x=w357) -> (.not. x?=w362:bool)
            n212 = Or(x=w374, y=w375) -> (x .or. y?=w372:bool)
            n213 = Compound Arithmetic op=OR(w386, w385, w375) -> (w352:bool)
            n214 = And(x=w363, y=w362) -> (x .and. y?=w361:bool)
            n215 = Compound Arithmetic op=OR(w388, w387, w374) -> (w354:bool)
            n216 = And(x=w372, y=w371) -> (x .and. y?=w373:bool)
            n217 = case shown="True" w361 {
              frame False {
              }
              frame True {
                n218 = property on="Iniciar / Finalizar" class="Bool (strict)"("Val(Sgnl)"=FALSE ("Value (Signaling)")) -> ()  [unwired: 2 in, 2 out]
              }
            }
            n219 = case shown="True" w373 {
              selector: w373 -> [_ w433]
              frame False {
              }
              frame True {
                n220 = property on="Iniciar / Finalizar" class="Bool (strict)"("Val(Sgnl)"=w433) -> ()  [unwired: 2 in, 2 out]
              }
            }
            n221 = property class="Bool (strict)"(reference=w358, "Value"=w352) -> ()  [unwired: 1 in, 2 out]
            n222 = property class="Bool (strict)"(reference=w359, "Value"=w354) -> ()  [unwired: 1 in, 2 out]
            n223 = case shown="False" w355 {
              tunnel: w354 -> [_ w408]
              tunnel: w352 -> [_ w407]
              tunnel: [TRUE w402] -> w335
              tunnel: w354 -> [w400 w406]
              tunnel: [w400 w405] -> w353
              tunnel: w352 -> [w399 w404]
              tunnel: [w399 w403] -> w351
              frame False {
              }
              frame True {
                n224 = Or(x=w408, y=w407) -> (x .or. y?=w409:bool)
                n225 = case shown="False" w409 {
                  tunnel: w406 -> [_ w415]
                  tunnel: [TRUE w415] -> w405
                  tunnel: w404 -> [_ w414]
                  tunnel: [FALSE w414] -> w403
                  tunnel: [FALSE TRUE] -> w402
                  frame False {
                  }
                  frame True {
                  }
                }
              }
            }
            n226 = Build Array(w353, w351, w357, w335, w322) -> (w334:bool[])
            n227 = case shown="True" w330 {
              tunnel: w335 -> [_ w396]
              tunnel: [w393 w395] -> w323
              tunnel: w334 -> [w393 _]
              tunnel: w322 -> [_ w394]
              frame False {
              }
              frame True {
                w398 = FALSE
                n228 = Build Array(w398, w398, TRUE ("element"), w396, w394) -> (w395:bool[])
              }
            }
            n229 = call-poly <vilib>:"DAQmx Write.vi"("task/channels in"=w384, "data"=w323, "error in"=w383) -> ("task out"=w381:refnum<k21>, "error out"=w382:errorcluster)  [unwired: 10 in, 1 out]
          }
        }
        n230 = property on="Stop" class="Bool (strict)"() -> ("Value"=w303:bool)  [unwired: 2 in, 2 out]
      }
      n231 = control-ref of="FactorsUnitatsPendents_D"() -> (w241:refnum<vi>)
      n232 = control-ref of="FactorsUnitatsPendents_F"() -> (w247:refnum<vi>)
      n233 = Initialize Array(0.0 ("element"), 3600 ("dimension size"), 2 ("dimension size")) -> (w203:dbl[][])
      n234 = control-ref of="IndexCel"() -> (w210:refnum<vi>)
      n235 = control-ref of="TaraF"() -> (w277:refnum<vi>)
      n236 = control-ref of="FSenseTara"() -> (w278:refnum<vi>)
      n237 = control-ref of="TablaFinal"() -> (w212:refnum<vi>)
      n238 = control-ref of="TaraD"() -> (w282:refnum<vi>)
      n239 = control-ref of="CaptadorF"() -> (w245:refnum<vi>)
      n240 = control-ref of="ParoProcessat"() -> (w229:refnum<vi>)
      n241 = while {
        shift-right: [w909] -> _
        shift-left: w203 -> [w908]
        tunnel: w288 -> [w907]
        tunnel: w290 -> [w896]
        tunnel: w239 -> [w906]
        tunnel: w289 -> [w905]
        tunnel: w287 -> [w903]
        tunnel: [w904] -> w243
        tunnel: w286 -> [w902]
        tunnel: w285 -> [w901]
        tunnel: w283 -> [w900]
        tunnel: w284 -> [w899]
        tunnel: w280 -> [w898]
        tunnel: w279 -> [w897]
        shift-right: [w895] -> _
        shift-left: FALSE ("ControlaCaigudaSortida") -> [w894]
        tunnel: w276 -> [w893]
        tunnel: w269 -> [w892]
        tunnel: w246 -> [w891]
        tunnel: w244 -> [w890]
        tunnel: w242 -> [w889]
        tunnel: w223 -> [w887]
        tunnel: w222 -> [w886]
        tunnel: w217 -> [w884]
        tunnel: w212 -> [w883]
        tunnel: w210 -> [w882]
        stop <- w888 stop-if-true
        n242 = property on="Procesa datos" class="Bool (strict)"() -> ("Value"=w885:bool)  [unwired: 2 in, 2 out]
        n243 = property on="Ensayo activo" class="Bool (strict)"("Value"=w885) -> ()  [unwired: 2 in, 2 out]
        n244 = event shown="[2] \"Guardar\": Value Change" {
          selector: w903 -> [_ _ _ _]
          dyn-events: [_ _ _ _] -> w904
          timeout: _ -> [_ _ _ _]
          tunnel: w908 -> [w958 w1081 w1143 _]
          tunnel: [w957 w1080 w1142 _] -> w909
          tunnel: w885 -> [w913 w1082 _ _]
          tunnel: w907 -> [w952 _ _ _]
          tunnel: w896 -> [w953 _ _ _]
          tunnel: w906 -> [w921 _ _ _]
          tunnel: w905 -> [w954 _ _ _]
          tunnel: w902 -> [w956 _ _ _]
          tunnel: w901 -> [w933 _ _ _]
          tunnel: w900 -> [w946 _ _ _]
          tunnel: w899 -> [w955 _ _ _]
          tunnel: w898 -> [w924 _ w1139 _]
          tunnel: w897 -> [w940 _ w1140 _]
          tunnel: [w951 _ _ _] -> w895
          tunnel: w894 -> [w950 _ _ _]
          tunnel: w893 -> [w949 _ w1137 _]
          tunnel: w892 -> [w935 _ _ _]
          tunnel: w891 -> [w939 _ w1135 _]
          tunnel: w890 -> [_ _ _ _]
          tunnel: w889 -> [w934 _ w1138 _]
          tunnel: w887 -> [w916 _ _ _]
          tunnel: w886 -> [w915 _ _ _]
          tunnel: w884 -> [_ w1079 _ w1166]
          tunnel: w883 -> [_ _ w1136 _]
          tunnel: w882 -> [w910 _ _ _]
          event User Event {
            n245 = event-data() -> ("DadesAdquirides"=w931:dbl[])  [unwired: 1 in, 3 out]
            n246 = property class="DigNum (strict)"(reference=w910) -> ("Value"=w911:u8)  [unwired: 1 in, 2 out]
            n247 = property on="Val. control sobrecarga" class="DigNum (strict)"() -> ("Value"=w937:dbl)  [unwired: 2 in, 2 out]
            n248 = Index Array(array=w931, index=w911) -> (element=w914:dbl)
            n249 = call "ConverteixAD.vi"("ValorSenseTara"=w954, "ValorAdquirid"=w914, "Unitats"=w940, "Tara"=w953, "FactorsUnitatsPendents"=w952) -> ("Escala"=w938:u8, "ValorActualAbs"=w948:dbl, "ValorSenseTara"=w945:dbl)  [unwired: 4 in]
            "ValorSenseTara" <- w945
            n250 = Absolute Value(x=w945) -> (abs(x)=w918:dbl)
            n251 = property on="CaptadorD" class="Ring (strict)"() -> ("Value"=w925:u16)  [unwired: 2 in, 2 out]
            n252 = call "FormatDades.vi"("Captador"=w939, "Escala"=w938, "ValorIn"=w948, "Unidades"=w940) -> ("NDecimals"=w936:u8, "ValorOut"=w947:dbl)  [unwired: 6 in]
            n253 = property on="Sobrecarga" class="Bool (strict)"() -> ("Value"=w944:bool)  [unwired: 2 in, 2 out]
            n254 = Greater?(x=w918, y=w937) -> (0:w941:bool)
            n255 = case shown="1" w925 {
              tunnel: [2 ("index") 3 ("index")] -> w927
              tunnel: w931 -> [w972 w973]
              tunnel: [w972 w973] -> w930
              frame 0, Default {
              }
              frame 1 {
              }
            }
            n256 = Not(x=w944) -> (.not. x?=w942:bool)
            n257 = And(x=w941, y=w942) -> (x .and. y?=w943:bool)
            n258 = property on="BtMaxF" class="Bool (strict)"() -> ("Value"=w932:bool)  [unwired: 2 in, 2 out]
            n259 = Index Array(array=w930, index=w927) -> (element=w929:dbl)
            n260 = call "ConverteixAD.vi"("ValorSenseTara"=w955, "ValorAdquirid"=w929, "Unitats"=w924, "Tara"=w946, "FactorsUnitatsPendents"=w956) -> ("ValorActualAbs"=w912:dbl)  [unwired: 4 in, 2 out]
            n261 = case shown="False" w943 {
              selector: w943 -> [_ w1075]
              tunnel: w941 -> [w1074 _]
              frame False {
                n262 = property on="Sobrecarga" class="Bool (strict)"("Value"=w1074) -> ()  [unwired: 2 in, 2 out]
              }
              frame True {
                n263 = property on="Sobrecarga" class="Bool (strict)"("Val(Sgnl)"=w1075) -> ()  [unwired: 2 in, 2 out]
              }
            }
            n264 = case shown="False" w932 {
              tunnel: w921 -> [w979 w983]
              tunnel: w947 -> [w978 w980]
              tunnel: w936 -> [w977 w985]
              tunnel: w935 -> [_ w984]
              tunnel: [w976 w982] -> w920
              tunnel: [w978 w980] -> w919
              tunnel: [w975 w980] -> w917
              frame False {
                n265 = property class="DigNum (strict)"(reference=w979, "Value"=w978, "Precision"=w977) -> (error out=w976:errorcluster, "Value"=w975:sgl)  [unwired: 1 in, 1 out]
              }
              frame True {
                n266 = property class="DigNum (strict)"(reference=w984) -> (error out=w986:errorcluster, "Value"=w981:sgl)  [unwired: 1 in, 1 out]
                n267 = property class="DigNum (strict)"(reference=w983, error in=w986, "Value"=w981, "Precision"=w985) -> (error out=w982:errorcluster)  [unwired: 1 out]
              }
            }
            n268 = property on="UnidadesD" class="Ring (strict)"() -> ("Value"=w923:u16)  [unwired: 2 in, 2 out]
            n269 = case shown="3" w927 {
              tunnel: [w964 w970] -> w928
              tunnel: [w959 w967] -> w926
              tunnel: w912 -> [w963 w969]
              tunnel: w925 -> [w960 w965]
              tunnel: w923 -> [w961 w966]
              frame 1, Default {
                n270 = call "FormatDefor.vi"("UnidadesD"=w961, "ValorIn"=w963, "CaptadorD"=w960, "ResoExten"=0 ("index")) -> ("ValorOut"=w964:dbl, "NDecimals"=w959:u8)  [unwired: 6 in]
              }
              frame 3 {
                n271 = property on="ResoExten" class="Ring (strict)"() -> ("Value"=w968:i8)  [unwired: 2 in, 2 out]
                n272 = call "FormatDefor.vi"("UnidadesD"=w966, "ValorIn"=w969, "CaptadorD"=w965, "ResoExten"=w968) -> ("ValorOut"=w970:dbl, "NDecimals"=w967:u8)  [unwired: 6 in]
              }
            }
            n273 = property class="DigNum (strict)"(reference=w933, "Value"=w928, "Precision"=w926) -> (error out=w922:errorcluster)  [unwired: 1 in, 1 out]
            n274 = case shown="True" w913 {
              tunnel: w958 -> [_ w1003]
              tunnel: [_ w1002] -> w957
              tunnel: [FALSE ("ControlaCaigudaSortida") w998] -> w951
              tunnel: w950 -> [_ w1004]
              tunnel: w949 -> [_ w1005]
              tunnel: w935 -> [_ w1001]
              tunnel: w933 -> [_ w1000]
              tunnel: w934 -> [_ w999]
              tunnel: w922 -> [_ w995]
              tunnel: w920 -> [_ w994]
              tunnel: w919 -> [_ w993]
              tunnel: w917 -> [_ w992]
              tunnel: w916 -> [_ w991]
              tunnel: w915 -> [_ w990]
              frame False {
                n275 = property on="ParaAssaig" class="Bool (strict)"("Value"=FALSE ("ParaAssaig")) -> ()  [unwired: 2 in, 2 out]
                n276 = property on="ParoRotura" class="Bool (strict)"("Value"=FALSE ("ParoRotura")) -> ()  [unwired: 2 in, 2 out]
              }
              frame True {
                n277 = property on="Precarga" class="Bool (strict)"() -> ("Value"=w997:bool)  [unwired: 2 in, 2 out]
                n278 = case shown="True" w997 {
                  selector: w997 -> [w1007 _]
                  tunnel: w993 -> [_ w1008]
                  tunnel: [w1006 w1010] -> w996
                  frame False {
                    n279 = Not(x=w1007) -> (.not. x?=w1006:bool)
                  }
                  frame True {
                    n280 = property on="PrecargaOn" class="Bool (strict)"() -> ("Value"=w1009:bool)  [unwired: 2 in, 2 out]
                    n281 = property on="ValorPrecarga" class="DigNum (strict)"() -> ("Value"=w1014:dbl)  [unwired: 2 in, 2 out]
                    n282 = Not(x=w1009) -> (.not. x?=w1013:bool)
                    n283 = Greater?(x=w1008, y=w1014) -> (0:w1011:bool)
                    n284 = And(x=w1013, y=w1011) -> (x .and. y?=w1012:bool)
                    n285 = case shown="False" w1012 {
                      selector: w1012 -> [_ w1017]
                      tunnel: [w1015 FALSE] -> w1010
                      tunnel: w1009 -> [w1015 _]
                      frame False {
                        n286 = property on="PrecargaOn" class="Bool (strict)"("Value"=w1015) -> ()  [unwired: 2 in, 2 out]
                      }
                      frame True {
                        n287 = property on="PrecargaOn" class="Bool (strict)"("Val(Sgnl)"=w1017) -> ()  [unwired: 2 in, 2 out]
                      }
                    }
                  }
                }
                n288 = case shown="True" w996 {
                  tunnel: [w1018 w1066] -> w998
                  tunnel: w1005 -> [_ w1065]
                  tunnel: w1004 -> [w1018 w1021]
                  tunnel: w1003 -> [w1019 w1064]
                  tunnel: [w1019 w1063] -> w1002
                  tunnel: w1001 -> [_ w1062]
                  tunnel: w1000 -> [_ w1061]
                  tunnel: w999 -> [_ w1060]
                  tunnel: w995 -> [_ w1046]
                  tunnel: w994 -> [_ _]
                  tunnel: w992 -> [_ w1037]
                  tunnel: w991 -> [_ w1042]
                  tunnel: w990 -> [_ w1029]
                  frame False {
                  }
                  frame True {
                    w1056 = 0
                    n289 = property class="DigNum (strict)"(reference=w1060) -> ("Value"=w1047:sgl)  [unwired: 1 in, 2 out]
                    n290 = property on="Valor de control sobrecarga" class="DigNum (strict)"() -> ("Value"=w1020:dbl)  [unwired: 2 in, 2 out]
                    n291 = property class="DigNum (strict)"(reference=w1042) -> (reference out=w1039:refnum<vi>, "Value"=w1041:dbl)  [unwired: 1 in, 1 out]
                    n292 = property class="DigNum (strict)"(reference=w1062) -> (reference out=w1050:refnum<vi>, "Value"=w1051:sgl)  [unwired: 1 in, 1 out]
                    n293 = property class="DigNum (strict)"(reference=w1029) -> ("Value"=w1036:sgl)  [unwired: 1 in, 2 out]
                    n294 = property class="DigNum (strict)"(reference=w1065) -> ("Value"=w1053:sgl)  [unwired: 1 in, 2 out]
                    n295 = property on="ActivaParoDefor" class="Bool (strict)"() -> ("Value"=w1043:bool)  [unwired: 2 in, 2 out]
                    n296 = Not Equal To 0?(x=w1047) -> (x != 0?=w1044:bool)
                    n297 = property class="DigNum (strict)"(reference=w1061, error in=w1046) -> ("Value"=w1048:sgl)  [unwired: 2 out]
                    n298 = property on="Fent_Rep" class="Bool (strict)"() -> ("Value"=w1023:bool)  [unwired: 2 in, 2 out]
                    n299 = And(x=w1043, y=w1044) -> (x .and. y?=w1024:bool)
                    n300 = Increment(x=w1041) -> (x+1=w1040:dbl)
                    n301 = Not(x=w1023) -> (.not. x?=w1022:bool)
                    n302 = property on="ParoDeforFet" class="Bool (strict)"() -> ("Value"=w1027:bool)  [unwired: 2 in, 2 out]
                    n303 = property on="ActivaParoCarga" class="Bool (strict)"() -> ("Value"=w1038:bool)  [unwired: 2 in, 2 out]
                    n304 = property on="ParoCargaFet" class="Bool (strict)"() -> ("Value"=w1033:bool)  [unwired: 2 in, 2 out]
                    n305 = Greater Or Equal?(x=w1037, y=w1036) -> (x >= y?=w1035:bool)
                    n306 = property class="DigNum (strict)"(reference=w1039, "Value"=w1040) -> ()  [unwired: 1 in, 2 out]
                    n307 = call "ControlFiAssaig.vi"("Actiu"=w1022, "PercentatgeCaiguda"=w1053, "FonsEscalaCaptador"=w1020, "ControlaCaigudaEntrada"=w1021, "ValorActual"=w1037, "ValorMaxim"=w1051) -> ("ControlaCaigudaSortida"=w1066:bool, "ParoRotura"=w1045:bool, "NouMaxim"=w1049:dbl)  [unwired: 3 in]
                    n308 = Not(x=w1027) -> (.not. x?=w1025:bool)
                    n309 = Not(x=w1033) -> (.not. x?=w1031:bool)
                    n310 = And(x=w1038, y=w1035) -> (x .and. y?=w1032:bool)
                    n311 = And(x=w1024, y=w1025) -> (x .and. y?=w1026:bool)
                    n312 = And(x=w1032, y=w1031) -> (x .and. y?=w1030:bool)
                    n313 = property class="DigNum (strict)"(reference=w1050, "Value"=w1049) -> ()  [unwired: 1 in, 2 out]
                    n314 = case shown="True" w1026 {
                      tunnel: w1047 -> [_ w1071]
                      tunnel: w1048 -> [_ w1070]
                      frame False {
                      }
                      frame True {
                        n315 = Greater?(x=w1070, y=w1071) -> (0:w1069:bool)
                        n316 = case shown="True" w1069 {
                          selector: w1069 -> [_ w1072]
                          frame False {
                          }
                          frame True {
                            n317 = property on="ParoDefor" class="Bool (strict)"("Val(Sgnl)"=w1072) -> ()  [unwired: 2 in, 2 out]
                          }
                        }
                      }
                    }
                    n318 = Array Size(array=w1064) -> (size(s)=w1057:i32[])
                    n319 = case shown="True" w1030 {
                      selector: w1030 -> [_ w1068]
                      frame False {
                      }
                      frame True {
                        n320 = property on="ParoCarga" class="Bool (strict)"("Val(Sgnl)"=w1068) -> ()  [unwired: 2 in, 2 out]
                      }
                    }
                    n321 = property on="ActivaParoRotura" class="Bool (strict)"() -> ("Value"=w1028:bool)  [unwired: 2 in, 2 out]
                    n322 = Index Array(array=w1057, index=w1056) -> (element=w1055:i32)
                    n323 = Equal?(x=w1055, y=w1056) -> (x = y?=w1054:bool)
                    n324 = And(x=w1028, y=w1045) -> (x .and. y?=w1034:bool)
                    n325 = call "Build XY Graph"("Reset"=w1054, "Y Input"=w1037, "X Input"=w1048) -> ("XY Graph"=→"?":cluster{"Y":dbl[], "Y":dbl[]}[])  [unwired: 7 in, 1 out]
                    n326 = Merge Signals(w1048, w1037) -> (w1058:dynamicdata)
                    n327 = case shown="True" w1034 {
                      selector: w1034 -> [_ w1073]
                      frame False {
                      }
                      frame True {
                        n328 = property on="ParoRotura" class="Bool (strict)"("Val(Sgnl)"=w1073) -> ()  [unwired: 2 in, 2 out]
                      }
                    }
                    n329 = property on="First time" class="Bool (strict)"("Value"=TRUE) -> ()  [unwired: 2 in, 2 out]
                    n330 = call "Convert from Dynamic Data"("Dynamic Data Type"=w1058) -> ("Array"=w1052:dbl[])  [unwired: 3 in]
                    n331 = Build Array (concatenate)(w1064, w1052) -> (w1063:dbl[][])
                    "Tabla" <- w1063
                  }
                }
              }
            }
          }
          event "Salir": Value Change {
            n332 = event-data() -> ()  [unwired: 1 in, 6 out]
            n333 = property on="rings" class="Arr (strict)"() -> ("Value"=w1078:refnum<vi>[])  [unwired: 2 in, 2 out]
            n334 = property on="Caselles" class="Arr (strict)"() -> ("Value"=w1077:refnum<vi>[])  [unwired: 2 in, 2 out]
            n335 = property on="Booleans" class="Arr (strict)"() -> ("Value"=w1076:refnum<vi>[])  [unwired: 2 in, 2 out]
            n336 = case shown="False" w1082 {
              selector: w1082 -> [_ w1110]
              tunnel: w1081 -> [_ w1112]
              tunnel: [_ w1112] -> w1080
              tunnel: w1079 -> [_ w1109]
              tunnel: w1078 -> [w1085 w1106]
              tunnel: w1077 -> [w1084 w1105]
              tunnel: w1076 -> [w1083 w1104]
              frame False {
                n337 = flat-sequence {
                  tunnel: w1085 -> [w1088]
                  tunnel: w1084 -> [w1087]
                  tunnel: w1083 -> [w1086]
                  frame #0 {
                    n338 = call "GuardaValorsPantalla.vi"("Rings"=w1088, "Caselles"=w1087, "Booleans"=w1086) -> ()  [unwired: 7 in, 1 out]
                  }
                  frame #1 {
                    n339 = call <vilib>:"DAQmx Stop Task.vi"("task/channels in"=refnum<k21> "USBAnalogIn") -> ("task out"=w1100:refnum<k21>, "error out"=w1099:errorcluster)  [unwired: 13 in]
                    n340 = call <vilib>:"DAQmx Stop Task.vi"("task/channels in"=refnum<k21> "USBAnalogOut") -> ("task out"=w1095:refnum<k21>, "error out"=w1097:errorcluster)  [unwired: 13 in]
                    n341 = call <vilib>:"DAQmx Stop Task.vi"("task/channels in"=refnum<k21> "USBDigitalIn") -> ("task out"=w1093:refnum<k21>, "error out"=w1094:errorcluster)  [unwired: 13 in]
                    n342 = call <vilib>:"DAQmx Stop Task.vi"("task/channels in"=refnum<k21> "USBEncoder") -> ("task out"=w1091:refnum<k21>)  [unwired: 13 in, 1 out]
                    n343 = call <vilib>:"DAQmx Stop Task.vi"("task/channels in"=refnum<k21> "USBDigitalOut") -> ("task out"=w1102:refnum<k21>, "error out"=w1101:errorcluster)  [unwired: 13 in]
                    n344 = call <vilib>:"DAQmx Clear Task.vi"("task in"=w1100, "error in"=w1099) -> ()  [unwired: 13 in, 1 out]
                    n345 = call <vilib>:"DAQmx Clear Task.vi"("task in"=w1095, "error in"=w1097) -> ()  [unwired: 13 in, 1 out]
                    n346 = call <vilib>:"DAQmx Clear Task.vi"("task in"=w1093, "error in"=w1094) -> ()  [unwired: 13 in, 1 out]
                    n347 = call <vilib>:"DAQmx Clear Task.vi"("task in"=w1102, "error in"=w1101) -> ()  [unwired: 13 in, 1 out]
                    n348 = call <vilib>:"DAQmx Clear Task.vi"("task in"=w1091) -> ()  [unwired: 14 in, 1 out]
                  }
                  frame #2 {
                    n349 = Quit LabVIEW(quit? (T)=TRUE) -> ()
                  }
                }
              }
              frame True {
                # "Mensaje de cancelar o no el ensayo activo"
                n350 = Index Array(array=w1109, index=2) -> (element=w1107:string)
                n351 = call "Display Message to User2"("Enable"=w1110, "Message"=w1107) -> ("OK"=w1111:bool)  [unwired: 8 in, 1 out]
                n352 = case shown="True" w1111 {
                  tunnel: w1106 -> [_ w1116]
                  tunnel: w1105 -> [_ w1115]
                  tunnel: w1104 -> [_ w1114]
                  frame False {
                    n353 = property on="Salir" class="Bool (strict)"("Value"=FALSE ("Salir")) -> ()  [unwired: 2 in, 2 out]
                  }
                  frame True {
                    n354 = flat-sequence {
                      tunnel: w1116 -> [w1119]
                      tunnel: w1115 -> [w1118]
                      tunnel: w1114 -> [w1117]
                      frame #0 {
                        n355 = call "GuardaValorsPantalla.vi"("Rings"=w1119, "Caselles"=w1118, "Booleans"=w1117) -> ()  [unwired: 7 in, 1 out]
                      }
                      frame #1 {
                        n356 = call <vilib>:"DAQmx Stop Task.vi"("task/channels in"=refnum<k21> "USBAnalogIn") -> ("task out"=w1131:refnum<k21>, "error out"=w1130:errorcluster)  [unwired: 13 in]
                        n357 = call <vilib>:"DAQmx Stop Task.vi"("task/channels in"=refnum<k21> "USBAnalogOut") -> ("task out"=w1126:refnum<k21>, "error out"=w1128:errorcluster)  [unwired: 13 in]
                        n358 = call <vilib>:"DAQmx Stop Task.vi"("task/channels in"=refnum<k21> "USBDigitalIn") -> ("task out"=w1124:refnum<k21>, "error out"=w1125:errorcluster)  [unwired: 13 in]
                        n359 = call <vilib>:"DAQmx Stop Task.vi"("task/channels in"=refnum<k21> "USBEncoder") -> ("task out"=w1122:refnum<k21>)  [unwired: 13 in, 1 out]
                        n360 = call <vilib>:"DAQmx Stop Task.vi"("task/channels in"=refnum<k21> "USBDigitalOut") -> ("task out"=w1133:refnum<k21>, "error out"=w1132:errorcluster)  [unwired: 13 in]
                        n361 = call <vilib>:"DAQmx Clear Task.vi"("task in"=w1131, "error in"=w1130) -> ()  [unwired: 13 in, 1 out]
                        n362 = call <vilib>:"DAQmx Clear Task.vi"("task in"=w1126, "error in"=w1128) -> ()  [unwired: 13 in, 1 out]
                        n363 = call <vilib>:"DAQmx Clear Task.vi"("task in"=w1124, "error in"=w1125) -> ()  [unwired: 13 in, 1 out]
                        n364 = call <vilib>:"DAQmx Clear Task.vi"("task in"=w1133, "error in"=w1132) -> ()  [unwired: 13 in, 1 out]
                        n365 = call <vilib>:"DAQmx Clear Task.vi"("task in"=w1122) -> ()  [unwired: 14 in, 1 out]
                      }
                      frame #2 {
                        n366 = Quit LabVIEW(quit? (T)=TRUE) -> ()
                      }
                    }
                  }
                }
              }
            }
          }
          event "Guardar": Value Change {
            n367 = event-data() -> ("NewVal"=w1141:bool)  [unwired: 1 in, 5 out]
            n368 = case shown="True" w1141 {
              tunnel: w1143 -> [w1144 w1163]
              tunnel: [w1144 w1162] -> w1142
              tunnel: w1140 -> [_ w1160]
              tunnel: w1139 -> [_ w1161]
              tunnel: w1138 -> [_ w1152]
              tunnel: w1137 -> [_ w1150]
              tunnel: [_ w1147] -> _
              tunnel: w1136 -> [_ w1147]
              tunnel: w1135 -> [_ w1145]
              frame False {
              }
              frame True {
                w1157 = ""
                n369 = property class="DigNum (strict)"(reference=w1152) -> ("Value"=w1151:sgl)  [unwired: 1 in, 2 out]
                n370 = property class="Arr (strict)"(reference=w1147) -> ("Value"=w1146:dbl[][])  [unwired: 1 in, 2 out]
                n371 = property class="DigNum (strict)"(reference=w1150) -> ("Value"=w1149:sgl)  [unwired: 1 in, 2 out]
                n372 = property on="ActivaParoDefor" class="Bool (strict)"() -> ("Value"=w1158:bool)  [unwired: 2 in, 2 out]
                n373 = property on="Velocidad Ensayo" class="DigNum (strict)"() -> ("Value"=w1159:sgl)  [unwired: 2 in, 2 out]
                n374 = property on="ValorPrecarga" class="DigNum (strict)"() -> ("Value"=w1148:dbl)  [unwired: 2 in, 2 out]
                n375 = property on="Nº Tests" class="DigNum (strict)"() -> ("Value"=w1153:u8)  [unwired: 2 in, 2 out]
                n376 = property on="ActivaParoRotura" class="Bool (strict)"() -> ("Value"=w1156:bool)  [unwired: 2 in, 2 out]
                n377 = property on="Precarga" class="Bool (strict)"() -> ("Value"=w1155:bool)  [unwired: 2 in, 2 out]
                n378 = call "CreaInformeExcel.vi"(0:w1160, 1:w1151, 2:w1157, 3:w1158, 4:w1159, 5:w1145, "Nom Assaig"=w1157, 7:w1155, "NºTests"=w1153, 9:w1148, 10:w1161, 11:w1156, "Tabla"=w1146, 13:w1149) -> ("status"=w1154:bool)  [unwired: 4 in, 1 out]
                n379 = case shown="False" w1154 {
                  tunnel: w1163 -> [w1164 _]
                  tunnel: [w1164 dbl[][] []] -> w1162
                  frame False {
                  }
                  frame True {
                  }
                }
              }
            }
          }
          event "BtEliminarUltima": Value Change {
            n380 = event-data() -> ("NewVal"=w1167:bool)  [unwired: 1 in, 5 out]
            n381 = case shown="True" w1167 {
              tunnel: w1166 -> [_ w1168]
              frame False {
              }
              frame True {
                n382 = property on="Nº Tests" class="DigNum (strict)"() -> ("Value"=w1169:u8)  [unwired: 2 in, 2 out]
                n383 = Greater Than 0?(x=w1169) -> (x > 0?=w1170:bool)
                n384 = case shown="True" w1170 {
                  tunnel: w1169 -> [_ w1178]
                  tunnel: w1168 -> [w1173 w1176]
                  frame False {
                    n385 = Index Array(array=w1173, index=4) -> (element=w1171:string)
                    n386 = call "Display Message to User3"("Message"=w1171) -> ()  [unwired: 9 in, 2 out]
                  }
                  frame True {
                    n387 = Index Array(array=w1176, index=3) -> (element=w1174:string)
                    n388 = call "Display Message to User6"("Message"=w1174) -> ("OK"=w1177:bool)  [unwired: 9 in, 1 out]
                    n389 = case shown="True" w1177 {
                      tunnel: w1178 -> [_ w1186]
                      frame False {
                      }
                      frame True {
                        w1189 = u8 2 ("y")
                        n390 = Subtract(x=w1186, y=1.0) -> (x-y=w1188:dbl)
                        n391 = Multiply(x=w1186, y=w1189) -> (x*y=w1190:u8)
                        n392 = property on="Tabla" class="Arr (strict)"() -> ("Number of Rows"=w1179:u32)  [unwired: 2 in, 2 out]
                        n393 = property on="TablaFinal" class="Arr (strict)"() -> ("Value"=w1182:dbl[][])  [unwired: 2 in, 2 out]
                        n394 = property on="Nº Tests" class="DigNum (strict)"("Value"=w1188) -> ()  [unwired: 2 in, 2 out]
                        n395 = Subtract(x=w1190, y=w1189) -> (x-y=w1180:u8)
                        n396 = property on="Columna" class="DigNum (strict)"("Value"=w1180) -> ()  [unwired: 2 in, 2 out]
                        n397 = Initialize Array(0.0 ("element"), 3600 ("dimension size"), 2 ("dimension size")) -> ()  [unwired: 1 out]
                        n398 = Delete From Array(array=w1182, length=w1179, index (col)=w1180) -> (array with subset deleted=w1181:dbl[][])  [unwired: 1 in, 1 out]
                        n399 = property on="TablaFinal" class="Arr (strict)"("Value"=w1181) -> ()  [unwired: 2 in, 2 out]
                      }
                    }
                  }
                }
              }
            }
          }
        }
        n400 = property on="Stop" class="Bool (strict)"() -> ("Value"=w888:bool)  [unwired: 2 in, 2 out]
      }
      n401 = control-ref of="NMostres"() -> (w215:refnum<vi>)
      n402 = control-ref of="Tabla"() -> (w213:refnum<vi>)
      n403 = control-ref of="ParoCargaFet"() -> (w216:refnum<vi>)
      n404 = control-ref of="ResetExten"() -> (w208:refnum<vi>)
      n405 = control-ref of="TablaFinal"() -> (w214:refnum<vi>)
      n406 = while {
        tunnel: w281 -> [w539]
        tunnel: w282 -> [w538]
        tunnel: w278 -> [w537]
        tunnel: w277 -> [w536]
        tunnel: w247 -> [w535]
        tunnel: w245 -> [w534]
        tunnel: w241 -> [w533]
        tunnel: w229 -> [w532]
        tunnel: w217 -> [w531]
        tunnel: w216 -> [w530]
        tunnel: w215 -> [w529]
        tunnel: w214 -> [w528]
        tunnel: w213 -> [w527]
        tunnel: w208 -> [w526]
        stop <- w540 stop-if-true
        n407 = event shown="[0] \"Iniciar / Finalizar\": Value Change" {
          selector: _ -> [_ _ _ _ _ _ _ _ _ _ _ _ _ _ _]
          dyn-events: _ -> [_ _ _ _ _ _ _ _ _ _ _ _ _ _ _]
          timeout: _ -> [_ _ _ _ _ _ _ _ _ _ _ _ _ _ _]
          tunnel: w539 -> [_ _ _ _ _ _ _ _ _ _ _ w854 _ _ w876]
          tunnel: w538 -> [_ _ _ _ _ _ w777 _ _ _ _ w851 _ _ w875]
          tunnel: w537 -> [_ _ _ _ _ _ _ _ _ _ _ _ _ w872 w874]
          tunnel: w536 -> [_ _ _ _ _ w761 _ _ _ _ _ _ _ w871 w873]
          tunnel: [_ _ _ _ _ _ _ _ _ w830 _ _ _ _ _] -> _
          tunnel: w535 -> [_ _ _ _ _ _ _ w796 _ w830 _ _ _ _ _]
          tunnel: w534 -> [_ _ _ _ _ w762 _ w792 _ _ _ _ _ _ _]
          tunnel: w533 -> [_ _ _ _ _ _ _ _ _ w829 _ _ _ _ _]
          tunnel: [_ _ _ _ _ _ _ _ _ _ _ w854 _ _ _] -> _
          tunnel: w532 -> [_ _ _ _ _ _ _ _ _ _ w836 _ _ _ _]
          tunnel: w531 -> [w544 w600 w618 w713 _ _ _ _ _ _ _ _ w857 _ _]
          tunnel: w530 -> [_ _ w616 _ _ _ _ _ _ _ _ _ _ _ _]
          tunnel: w529 -> [w543 _ _ _ _ _ _ _ _ _ _ _ _ _ _]
          tunnel: w528 -> [w542 w599 _ _ _ _ _ _ _ _ _ _ _ _ _]
          tunnel: w527 -> [w541 w598 _ _ _ _ _ _ _ _ _ _ _ _ _]
          tunnel: w526 -> [_ _ _ _ _ _ _ _ _ _ _ _ w859 _ _]
          event "Iniciar / Finalizar": Value Change {
            n408 = event-data() -> ()  [unwired: 1 in, 5 out]
            n409 = property on="Iniciar / Finalizar" class="Bool (strict)"() -> ("Value"=w545:bool)  [unwired: 2 in, 2 out]
            n410 = case shown="False" w545 {
              tunnel: w544 -> [_ w594]
              tunnel: w543 -> [w551 _]
              tunnel: w542 -> [w548 _]
              tunnel: w541 -> [w547 _]
              tunnel: w541 -> [w546 _]
              frame False {
                n411 = flat-sequence {
                  tunnel: w551 -> [w557]
                  tunnel: [w555] -> w549
                  tunnel: w548 -> [w554]
                  tunnel: w547 -> [w553]
                  tunnel: [w580] -> w550
                  tunnel: w549 -> [w580]
                  tunnel: w550 -> [w588]
                  tunnel: [w586] -> _
                  tunnel: w546 -> [w586]
                  frame #0 {
                    w558 = FALSE ("ParoCarga")
                    n412 = property on="ParoCarga" class="Bool (strict)"("Value"=w558) -> ()  [unwired: 2 in, 2 out]
                    n413 = property on="ParoCargaFet" class="Bool (strict)"("Value"=w558) -> ()  [unwired: 2 in, 2 out]
                    n414 = property on="ParoDefor" class="Bool (strict)"("Value"=w558) -> ()  [unwired: 2 in, 2 out]
                    n415 = property on="ParoDeforFet" class="Bool (strict)"("Value"=w558) -> ()  [unwired: 2 in, 2 out]
                    n416 = property on="Procesa datos" class="Bool (strict)"("Value"=FALSE) -> ()  [unwired: 2 in, 2 out]
                    n417 = property on="ParaAssaig" class="Bool (strict)"("Value"=TRUE ("ParaAssaig")) -> ()  [unwired: 2 in, 2 out]
                    n418 = property on="Mante_a_Vel_0" class="Bool (strict)"("Value"=FALSE ("Mante_a_Vel_0")) -> ()  [unwired: 2 in, 2 out]
                    n419 = property on="First time" class="Bool (strict)"() -> ("Value"=w556:bool)  [unwired: 2 in, 2 out]
                    n420 = case shown="True" w556 {
                      tunnel: [_ w569] -> _
                      tunnel: w557 -> [_ w569]
                      tunnel: [_ w567] -> w555
                      tunnel: w554 -> [_ w566]
                      tunnel: w553 -> [_ w562]
                      frame False {
                      }
                      frame True {
                        n421 = property class="DigNum (strict)"(reference=w569) -> (reference out=w567:refnum<vi>, "Value"=w568:dbl)  [unwired: 1 in, 1 out]
                        n422 = property on="Nº Tests" class="DigNum (strict)"() -> ("Value"=w574:u8)  [unwired: 2 in, 2 out]
                        n423 = property on="ArraiMostresxProva" class="Arr (strict)"() -> ("Value"=w575:dbl[])  [unwired: 2 in, 2 out]
                        n424 = Increment(x=w574) -> (x+1=w576:u8)
                        n425 = property on="Nº Tests" class="DigNum (strict)"("Value"=w576) -> ()  [unwired: 2 in, 2 out]
                        n426 = Insert Into Array(array=w575, index=w574, new element=w568) -> (w573:dbl[])
                        n427 = property on="ArraiMostresxProva" class="Arr (strict)"("Value"=w573) -> ()  [unwired: 2 in, 2 out]
                        n428 = property on="StringsEstatMáquina" class="Arr (strict)"() -> ("Value"=w572:string[])  [unwired: 2 in, 2 out]
                        n429 = property on="CodiAturada" class="DigNum (strict)"() -> ("Value"=w570:u32)  [unwired: 2 in, 2 out]
                        n430 = property class="Arr (strict)"(reference=w562) -> ("Value"=w561:dbl[][])  [unwired: 1 in, 2 out]
                        n431 = property class="Arr (strict)"(reference=w566) -> (reference out=w564:refnum<vi>, "Value"=w565:dbl[][])  [unwired: 1 in, 1 out]
                        n432 = Index Array(array=w572, index=w570) -> (element=w571:string)
                        n433 = property on="Columna" class="DigNum (strict)"() -> ("Value"=w577:i32)  [unwired: 2 in, 2 out]
                        n434 = property on="Estado ensayo:" class="Str"("Value"=w571) -> ()  [unwired: 2 in, 2 out]
                        n435 = Add(x=w577, y=2) -> (x+y=w578:i32)
                        n436 = Insert Into Array(array=w565, index (col)=w577, new element=w561) -> (w563:dbl[][])  [unwired: 1 in]
                        n437 = property on="Columna" class="DigNum (strict)"("Value"=w578) -> ()  [unwired: 2 in, 2 out]
                        n438 = property class="Arr (strict)"(reference=w564, "Value"=w563) -> ()  [unwired: 1 in, 2 out]
                      }
                    }
                  }
                  frame #1 {
                    n439 = Wait (ms)(milliseconds to wait=u32 200) -> ()  [unwired: 1 out]
                  }
                  frame #2 {
                    n440 = property class="DigNum (strict)"(reference=w588, "Value"=0.0 ("NMostres")) -> ()  [unwired: 1 in, 2 out]
                    n441 = Initialize Array(0.0 ("element"), 3600 ("dimension size"), 2 ("dimension size")) -> (w582:dbl[][])
                    n442 = property on="Rep. Fetes" class="DigNum (strict)"("Value"=u8 0 ("Rep. Fetes")) -> ()  [unwired: 2 in, 2 out]
                    n443 = property class="Arr (strict)"(reference=w586, "Value"=w582) -> ()  [unwired: 1 in, 2 out]
                    n444 = property on="PrecargaOn" class="Bool (strict)"("Value"=FALSE ("PrecargaOn")) -> ()  [unwired: 2 in, 2 out]
                    n445 = property on="First time" class="Bool (strict)"("Value"=FALSE) -> ()  [unwired: 2 in, 2 out]
                  }
                }
              }
              frame True {
                n446 = Index Array(array=w594, index=18) -> (element=w593:string)
                n447 = property on="Estado ensayo:" class="Str"("Value"=w593) -> ()  [unwired: 2 in, 2 out]
                n448 = property on="Maxim" class="DigNum (strict)"("Value"=0.0 ("Maxim")) -> (error out=w595:errorcluster)  [unwired: 2 in, 1 out]
                n449 = property on="Procesa datos" class="Bool (strict)"(error in=w595, "Value"=TRUE) -> ()  [unwired: 1 in, 2 out]
              }
            }
          }
          event "Ensayonuevo": Value Change {
            n450 = event-data() -> ("NewVal"=w601:bool)  [unwired: 1 in, 5 out]
            n451 = case shown="True" w601 {
              tunnel: w600 -> [_ w606]
              tunnel: [_ w603] -> _
              tunnel: w599 -> [_ w603]
              tunnel: w598 -> [_ w602]
              frame False {
              }
              frame True {
                n452 = Index Array(array=w606, index=0) -> (element=w604:string)
                n453 = call "Display Message to User"("Message"=w604) -> ("OK"=w607:bool)  [unwired: 9 in, 1 out]
                n454 = case shown="True" w607 {
                  tunnel: w603 -> [_ w610]
                  tunnel: w602 -> [_ w609]
                  frame False {
                  }
                  frame True {
                    (unwired) dbl[][] [] ("Value")
                    (unwired) dbl[][] [] ("TablaFinal")
                    n455 = property on="Columna" class="DigNum (strict)"("Value"=0 ("Columna")) -> ()  [unwired: 2 in, 2 out]
                    n456 = Initialize Array(0.0 ("element"), 3600 ("dimension size"), 2 ("dimension size")) -> (w608:dbl[][])
                    n457 = property on="Nº Tests" class="DigNum (strict)"("Value"=u8 0 ("Nº Tests")) -> ()  [unwired: 2 in, 2 out]
                    n458 = property class="Arr (strict)"(reference=w610, "Value"=w608) -> ()  [unwired: 1 in, 2 out]
                    n459 = property class="Arr (strict)"(reference=w609, "Value"=w608) -> ()  [unwired: 1 in, 2 out]
                  }
                }
              }
            }
          }
          event "ParoCarga": Value Change {
            n460 = event-data() -> ("NewVal"=w617:bool)  [unwired: 1 in, 5 out]
            n461 = case shown="True" w617 {
              tunnel: w618 -> [_ w622]
              tunnel: w616 -> [_ w621]
              frame False {
              }
              frame True {
                n462 = property class="Bool (strict)"(reference=w621) -> (reference out=w619:refnum<vi>, "Value"=w620:bool)  [unwired: 1 in, 1 out]
                n463 = case shown="False" w620 {
                  tunnel: w622 -> [w623 _]
                  tunnel: w619 -> [w626 _]
                  frame False {
                    n464 = property on="FinalEnsayo" class="Bool (strict)"() -> (error out=w625:errorcluster, "Value"=w634:bool)  [unwired: 2 in, 1 out]
                    n465 = property class="Bool (strict)"(reference=w626, error in=w625, "Value"=TRUE ("ParoCargaFet")) -> (reference out=w624:refnum<vi>, error out=w628:errorcluster)
                    n466 = Index Array(array=w623, index=1) -> (element=w630:string)
                    n467 = case shown="False" w634 {
                      tunnel: [w646 FALSE ("SI")] -> w635
                      tunnel: [w641 w705] -> w632
                      tunnel: w630 -> [w645 _]
                      tunnel: w628 -> [w640 w705]
                      tunnel: w624 -> [w639 _]
                      tunnel: w623 -> [w636 _]
                      frame False {
                        n468 = property on="Rep. A Fer" class="DigNum (strict)"() -> ("Value"=w644:sgl)  [unwired: 2 in, 2 out]
                        n469 = Index Array(array=w636, index=5) -> (element=w637:string)
                        n470 = Greater?(x=w644, y=u8 0) -> (0:w642:bool)
                        n471 = case shown="True" w642 {
                          tunnel: [w667 w703] -> w646
                          tunnel: w645 -> [w657 w702]
                          tunnel: w644 -> [w666 _]
                          tunnel: w640 -> [w663 w701]
                          tunnel: [w662 w701] -> w641
                          tunnel: w639 -> [w661 _]
                          tunnel: w637 -> [w654 _]
                          tunnel: w636 -> [w651 _]
                          frame True {
                            n472 = property on="Rep. Fetes" class="DigNum (strict)"() -> ("Value"=w664:u8)  [unwired: 2 in, 2 out]
                            n473 = Index Array(array=w651, index=6) -> (element=w648:string)
                            n474 = Index Array(array=w651, index=7) -> (element=w647:string)
                            n475 = Increment(x=w664) -> (x+1=w656:u8)
                            n476 = property on="Fent_Rep" class="Bool (strict)"("Value"=TRUE ("Fent_Rep")) -> ()  [unwired: 2 in, 2 out]
                            n477 = Greater Or Equal?(x=w656, y=w666) -> (x >= y?=w665:bool)
                            n478 = Format Into String(w656) -> (resulting string=w653:string)  [unwired: 3 in, 1 out]
                            n479 = Concatenate Strings(w654, w653) -> (w655:string)
                            n480 = Concatenate Strings(w655, "\r", w657) -> (w652:string)
                            n481 = case shown="True" w665 {
                              tunnel: [w670 w688] -> w667
                              tunnel: w656 -> [w677 w692]
                              tunnel: w663 -> [w678 _]
                              tunnel: [w678 w695] -> w662
                              tunnel: w661 -> [_ w694]
                              tunnel: [w677 w692] -> w660
                              tunnel: w652 -> [w673 w691]
                              tunnel: w648 -> [w669 w685]
                              tunnel: w647 -> [w668 w684]
                              frame True {
                                n482 = call <vilib>:"Three Button Dialog.vi"("Allow user to close window? (TRUE)"=FALSE, "Right Button Text (\"Cancel\")"=w668, "Left Button Text (\"Yes\")"=w669, "message"=w673) -> ("Which Button?"=w674:T6)  [unwired: 7 in]
                                n483 = case shown="\"Right Button\"" w674 {
                                tunnel: [TRUE w681 TRUE] -> w670
                                tunnel: [FALSE w681 TRUE ("Mante_a_Vel_0")] -> w672
                                frame "Left Button", Default {
                                }
                                frame "Center Button" {
                                w681 = FALSE
                                }
                                frame "Right Button" {
                                }
                                }
                                n484 = property on="Mante_a_Vel_0" class="Bool (strict)"("Value"=w672) -> (error out=w671:errorcluster)  [unwired: 2 in, 1 out]
                                n485 = property on="Fent_Rep" class="Bool (strict)"(error in=w671, "Value"=FALSE ("Fent_Rep")) -> ()  [unwired: 1 in, 2 out]
                              }
                              frame False {
                                n486 = call <vilib>:"Three Button Dialog.vi"("Allow user to close window? (TRUE)"=FALSE, "Right Button Text (\"Cancel\")"=w684, "Left Button Text (\"Yes\")"=w685, "message"=w691) -> ("Which Button?"=w689:T6)  [unwired: 7 in]
                                n487 = case shown="\"Right Button\"" w689 {
                                tunnel: [TRUE w698 TRUE] -> w688
                                tunnel: [FALSE w698 TRUE ("Mante_a_Vel_0")] -> w687
                                frame "Left Button", Default {
                                }
                                frame "Center Button" {
                                w698 = FALSE
                                }
                                frame "Right Button" {
                                }
                                }
                                n488 = property on="Mante_a_Vel_0" class="Bool (strict)"("Value"=w687) -> (error out=w686:errorcluster)  [unwired: 2 in, 1 out]
                                n489 = property class="Bool (strict)"(reference=w694, error in=w686, "Value"=FALSE) -> (error out=w695:errorcluster)  [unwired: 1 out]
                              }
                            }
                            n490 = property on="Rep. Fetes" class="DigNum (strict)"("Value"=w660) -> ()  [unwired: 2 in, 2 out]
                          }
                          frame False {
                            n491 = call "Display Message to User7"("Message"=w702) -> ("SI"=w703:bool)  [unwired: 9 in, 1 out]
                          }
                        }
                      }
                      frame True {
                      }
                    }
                    n492 = case shown="True" w635 {
                      tunnel: w632 -> [w708 w712]
                      tunnel: [w708 w712] -> w629
                      frame False {
                        n493 = property on="Procesa datos" class="Bool (strict)"("Value"=FALSE ("Procesa datos")) -> (error out=w710:errorcluster)  [unwired: 2 in, 1 out]
                        n494 = property on="Iniciar / Finalizar" class="Bool (strict)"(error in=w710, "Val(Sgnl)"=FALSE ("Value (Signaling)")) -> (error out=w706:errorcluster)  [unwired: 1 in, 1 out]
                        n495 = property on="Rep. Fetes" class="DigNum (strict)"(error in=w706, "Value"=u8 0 ("Rep. Fetes")) -> ()  [unwired: 1 in, 2 out]
                      }
                      frame True {
                      }
                    }
                    n496 = property on="ParoCarga" class="Bool (strict)"(error in=w629, "Value"=FALSE ("ParoCarga")) -> ()  [unwired: 1 in, 2 out]
                  }
                  frame True {
                  }
                }
              }
            }
          }
          event "ParoDefor": Value Change {
            n497 = event-data() -> ("NewVal"=w714:bool)  [unwired: 1 in, 5 out]
            n498 = case shown="True" w714 {
              tunnel: w713 -> [_ w715]
              frame False {
              }
              frame True {
                n499 = property on="ParoDeforFet" class="Bool (strict)"() -> (error out=w717:errorcluster, "Value"=w716:bool)  [unwired: 2 in, 1 out]
                n500 = case shown="False" w716 {
                  tunnel: w717 -> [w727 _]
                  tunnel: w715 -> [w720 _]
                  frame False {
                    n501 = property on="FinalEnsayo" class="Bool (strict)"(error in=w727) -> (error out=w725:errorcluster, "Value"=w728:bool)  [unwired: 1 in, 1 out]
                    n502 = property on="ParoDeforFet" class="Bool (strict)"(error in=w725, "Value"=TRUE ("ParoCargaFet")) -> (error out=w724:errorcluster)  [unwired: 1 in, 1 out]
                    n503 = Index Array(array=w720, index=1) -> (element=w718:string)
                    n504 = case shown="False" w728 {
                      tunnel: [w732 FALSE ("SI")] -> w729
                      tunnel: w724 -> [w731 w733]
                      tunnel: [w731 w733] -> w726
                      tunnel: w718 -> [w730 _]
                      frame False {
                        n505 = call "Display Message to User4"("Message"=w730) -> ("SI"=w732:bool)  [unwired: 9 in, 1 out]
                      }
                      frame True {
                      }
                    }
                    n506 = case shown="False" w729 {
                      tunnel: w726 -> [w735 w739]
                      tunnel: [w735 w739] -> w721
                      frame False {
                        n507 = property on="Procesa datos" class="Bool (strict)"("Value"=FALSE ("Procesa datos")) -> (error out=w737:errorcluster)  [unwired: 2 in, 1 out]
                        n508 = property on="Iniciar / Finalizar" class="Bool (strict)"(error in=w737, "Val(Sgnl)"=FALSE ("Value (Signaling)")) -> ()  [unwired: 1 in, 2 out]
                      }
                      frame True {
                      }
                    }
                    n509 = property on="ParoDefor" class="Bool (strict)"(error in=w721, "Value"=FALSE ("ParoCarga")) -> ()  [unwired: 1 in, 2 out]
                  }
                  frame True {
                  }
                }
              }
            }
          }
          event "ParoRotura": Value Change {
            n510 = event-data() -> ("NewVal"=w740:bool)  [unwired: 1 in, 5 out]
            n511 = case shown="True" w740 {
              frame False {
              }
              frame True {
                n512 = property on="Procesa datos" class="Bool (strict)"("Value"=FALSE ("Procesa datos")) -> (error out=w742:errorcluster)  [unwired: 2 in, 1 out]
                n513 = property on="Iniciar / Finalizar" class="Bool (strict)"(error in=w742, "Val(Sgnl)"=FALSE ("Value (Signaling)")) -> ()  [unwired: 1 in, 2 out]
              }
            }
          }
          event "UnidadesF": Value Change {
            n514 = event-data() -> ("NewVal"=w749:u16)  [unwired: 1 in, 5 out]
            n515 = property class="Ring (strict)"(reference=w762) -> ("Strings []"=w747:string[], "RingText.Text"=w746:string)  [unwired: 1 in, 2 out]
            n516 = Search 1D Array(1D array=w747, element=w746) -> (index of element=w748:i32)  [unwired: 1 in]
            n517 = property on="ConversioUnitatsF" class="Arr (strict)"() -> ("Value"=w763:dbl[])  [unwired: 2 in, 2 out]
            n518 = property class="DigNum (strict)"(reference=w761, "Value"=sgl 0.0) -> ()  [unwired: 1 in, 2 out]
            n519 = case shown="0, Default" w748 {
              tunnel: [w765 w766] -> w759
              frame 0, Default {
                n520 = property on="ValorSobrecargaC1" class="DigNum (strict)"() -> ("Value"=w765:dbl)  [unwired: 2 in, 2 out]
              }
              frame 1 {
                n521 = property on="ValorSobrecargaC2" class="DigNum (strict)"() -> ("Value"=w766:dbl)  [unwired: 2 in, 2 out]
              }
            }
            n522 = property on="UnidadesF" class="Ring (strict)"("Value"=w749) -> ()  [unwired: 2 in, 2 out]
            n523 = Index Array(array=w763, index=w749) -> (element=w764:dbl)
            n524 = property on="PerCentPrecarga" class="DigNum (strict)"() -> ("Value"=w745:sgl)  [unwired: 2 in, 2 out]
            n525 = Multiply(x=w759, y=w764) -> (x*y=w755:dbl)
            n526 = Multiply(x=w755, y=w745) -> (x*y=w758:dbl)
            n527 = Divide(x=w758, y=100.0) -> (x/y=w756:dbl)
            n528 = property on="Valor de control sobrecarga" class="DigNum (strict)"("Value"=w755) -> ()  [unwired: 2 in, 2 out]
            n529 = property on="ArraiUnitats" class="Arr (strict)"() -> ("Value"=w754:cluster{"String":string, "Value":u16}[])  [unwired: 2 in, 2 out]
            n530 = property on="ValorPrecarga" class="DigNum (strict)"("Value"=w756) -> ()  [unwired: 2 in, 2 out]
            n531 = Index Array(array=w754, index=w749) -> (element=w753:cluster{"String":string, "Value":u16})
            n532 = Unbundle By Name(w753) -> ("String"=w750:string)
            n533 = property on="Fuerza" class="DigNum (strict)"() -> ("Caption.Text"=w744:string)  [unwired: 2 in, 2 out]
            n534 = Concatenate Strings(w744, " - " ("string"), w750) -> (w752:string)
            n535 = property class="XYGraph (strict)"("YScale.NameLbl.Text"=w752) -> ()  [unwired: 2 in, 2 out]
          }
          event "UnidadesD": Value Change {
            n536 = event-data() -> ("NewVal"=w772:u16)  [unwired: 1 in, 5 out]
            n537 = property class="DigNum (strict)"(reference=w777, "Value"=sgl 0.0) -> ()  [unwired: 1 in, 2 out]
            n538 = property on="UnidadesD" class="Ring (strict)"() -> ("StringsAndValues[]"=w773:T7)  [unwired: 2 in, 2 out]
            n539 = property class="XYGraph (strict)"() -> ("XScale.NameLbl.Text"=w775:string)  [unwired: 2 in, 2 out]
            n540 = Index Array(array=w773, index=w772) -> (element=w770:cluster{"String":string, "Value":u16})
            n541 = Unbundle By Name(w770) -> ("String"=w768:string)
            n542 = Match Pattern(string=w775, regular expression="-") -> (before substring=w771:string)  [unwired: 1 in, 3 out]
            n543 = Concatenate Strings(w771, "- " ("regular expression"), w768) -> (w769:string)
            n544 = property class="XYGraph (strict)"("XScale.NameLbl.Text"=w769) -> ()  [unwired: 2 in, 2 out]
          }
          event "CaptadorF": Value Change {
            # "Quan està carregant la darrera configuració no reinicia les unitats"
            n545 = event-data() -> ()  [unwired: 1 in, 6 out]
            n546 = property class="Ring (strict)"(reference=w792) -> ("Strings []"=w794:string[], "RingText.Text"=w793:string)  [unwired: 1 in, 2 out]
            n547 = Search 1D Array(1D array=w794, element=w793) -> (index of element=w791:i32)  [unwired: 1 in]
            "IndexCel" <- w791
            n548 = Equal?(x=w791, y=0) -> (x = y?=w795:bool)
            n549 = case shown="True" w795 {
              tunnel: [w807 w809] -> w779
              tunnel: [w808 w811] -> w782
              tunnel: [1 ("index") 0 ("index")] -> w785
              frame False {
                n550 = property on="ValorSobrecargaC2" class="DigNum (strict)"() -> ("Value"=w808:dbl)  [unwired: 2 in, 2 out]
                n551 = property on="UnidadesF_C2" class="Ring (strict)"() -> ("StringsAndValues[]"=w807:T7)  [unwired: 2 in, 2 out]
              }
              frame True {
                n552 = property on="UnidadesF_C1" class="Ring (strict)"() -> ("StringsAndValues[]"=w809:T7)  [unwired: 2 in, 2 out]
                n553 = property on="ValorSobrecargaC1" class="DigNum (strict)"() -> ("Value"=w811:dbl)  [unwired: 2 in, 2 out]
              }
            }
            n554 = property on="ConversioUnitatsF" class="Arr (strict)"() -> ("Value"=w788:dbl[])  [unwired: 2 in, 2 out]
            n555 = property on="Calibratge" class="Arr (strict)"() -> ("Value"=w789:dbl[])  [unwired: 2 in, 2 out]
            n556 = Index Array(array=w789, index=w785) -> (element=w787:dbl)
            n557 = Multiply(x=w788, y=w787) -> (x*y=w786:dbl[])
            n558 = property class="Arr (strict)"(reference=w796, "Value"=w786) -> ()  [unwired: 1 in, 2 out]
            n559 = property on="CarregaConfig" class="Bool (strict)"() -> ("Value"=w778:bool)  [unwired: 2 in, 2 out]
            n560 = property on="PerCentPrecarga" class="DigNum (strict)"() -> ("Value"=w780:sgl)  [unwired: 2 in, 2 out]
            n561 = property on="Valor de control sobrecarga" class="DigNum (strict)"("Value"=w782) -> ()  [unwired: 2 in, 2 out]
            n562 = case shown="True" w778 {
              tunnel: w779 -> [w800 w801]
              frame False {
                n563 = Index Array(array=w800, index=0) -> (element=w798:cluster{"String":string, "Value":u16})
                n564 = Unbundle By Name(w798) -> ("Value"=w797:u16)
                n565 = property on="UnidadesF" class="Ring (strict)"("StringsAndValues[]"=w800, "Val(Sgnl)"=w797) -> ()  [unwired: 2 in, 2 out]
              }
              frame True {
                n566 = property on="UnidadesF" class="Ring (strict)"("StringsAndValues[]"=w801) -> (error out=w803:errorcluster, "Value"=w802:u16)  [unwired: 2 in, 1 out]
                n567 = property on="CarregaConfig" class="Bool (strict)"(error in=w803, "Value"=FALSE ("CarregaConfig")) -> (error out=w804:errorcluster)  [unwired: 1 in, 1 out]
                n568 = property on="UnidadesF" class="Ring (strict)"(error in=w804, "Val(Sgnl)"=w802) -> ()  [unwired: 1 in, 2 out]
              }
            }
            n569 = Multiply(x=w782, y=w780) -> (x*y=w784:dbl)
            n570 = Divide(x=w784, y=100.0) -> (x/y=w781:dbl)
            n571 = property on="ValorPrecarga" class="DigNum (strict)"("Value"=w781) -> ()  [unwired: 2 in, 2 out]
          }
          event "PerCentPrecarga": Value Change {
            n572 = event-data() -> ("NewVal"=w814:sgl)  [unwired: 1 in, 5 out]
            n573 = property on="Valor de control sobrecarga" class="DigNum (strict)"() -> ("Value"=w813:dbl)  [unwired: 2 in, 2 out]
            n574 = Multiply(x=w813, y=w814) -> (x*y=w816:dbl)
            n575 = Divide(x=w816, y=100.0) -> (x/y=w812:dbl)
            n576 = property on="ValorPrecarga" class="DigNum (strict)"("Value"=w812) -> ()  [unwired: 2 in, 2 out]
          }
          event "CaptadorD": Value Change {
            n577 = event-data() -> ("NewVal"=w825:u16)  [unwired: 1 in, 5 out]
            n578 = property on="Calibratge D" class="Arr (strict)"() -> ("Value"=w827:dbl[])  [unwired: 2 in, 2 out]
            n579 = property on="ConversioUnitatsD" class="Arr (strict)"() -> ("Value"=w828:dbl[])  [unwired: 2 in, 2 out]
            n580 = Index Array(array=w827, index=w825) -> (element=w832:dbl)
            n581 = Multiply(x=w828, y=w832) -> (x*y=w831:dbl[])
            n582 = property on="UnidadesD" class="Ring (strict)"() -> ("Value"=w823:u16, "StringsAndValues[]"=w822:T7)  [unwired: 2 in, 2 out]
            n583 = property on="CaptadorD" class="Ring (strict)"() -> ("StringsAndValues[]"=w826:T7)  [unwired: 2 in, 2 out]
            n584 = property class="Arr (strict)"(reference=w829, "Value"=w831) -> ()  [unwired: 1 in, 2 out]
            n585 = Index Array(array=w826, index=w825) -> (element=w824:cluster{"String":string, "Value":u16})
            n586 = Index Array(array=w822, index=w823) -> (element=w821:cluster{"String":string, "Value":u16})
            n587 = Unbundle By Name(w824) -> ("String"=w819:string)
            n588 = Unbundle By Name(w821) -> ("String"=w817:string)
            n589 = Concatenate Strings(w819, " - " ("string"), w817) -> (w820:string)
            n590 = property class="XYGraph (strict)"("XScale.NameLbl.Text"=w820) -> ()  [unwired: 2 in, 2 out]
          }
          event "Paro Emergencia", "Sobrecarga": Value Change {
            n591 = event-data() -> ("NewVal"=w837:bool)  [unwired: 1 in, 5 out]
            n592 = property on="StringsEstatMáquina" class="Arr (strict)"() -> ("Value"=w834:string[])  [unwired: 2 in, 2 out]
            n593 = property on="CodiAturada" class="DigNum (strict)"() -> ("Value"=w833:u32)  [unwired: 2 in, 2 out]
            n594 = case shown="True" w837 {
              tunnel: [w839 w843] -> w835
              tunnel: w836 -> [_ w848]
              tunnel: w834 -> [w840 w842]
              tunnel: w833 -> [w838 w841]
              frame False {
                n595 = Index Array(array=w840, index=w838) -> (element=w839:string)
              }
              frame True {
                n596 = property on="ParoProcessat" class="Bool (strict)"(reference=w848, "Value"=TRUE) -> ()  [unwired: 1 in, 2 out]
                n597 = property on="Procesa datos" class="Bool (strict)"("Value"=FALSE ("Procesa datos")) -> (error out=w846:errorcluster)  [unwired: 2 in, 1 out]
                n598 = property on="Iniciar / Finalizar" class="Bool (strict)"() -> ("Value"=w844:bool)  [unwired: 2 in, 2 out]
                n599 = Index Array(array=w842, index=w841) -> (element=w843:string)
                n600 = case shown="True" w844 {
                  tunnel: w846 -> [_ w850]
                  frame False {
                  }
                  frame True {
                    n601 = property on="Iniciar / Finalizar" class="Bool (strict)"(error in=w850, "Val(Sgnl)"=FALSE ("Value (Signaling)")) -> ()  [unwired: 1 in, 2 out]
                  }
                }
              }
            }
            n602 = property on="Estado ensayo:" class="Str"("Value"=w835) -> ()  [unwired: 2 in, 2 out]
          }
          event "BtTaraD": Value Change {
            n603 = event-data() -> ()  [unwired: 1 in, 6 out]
            n604 = property class="DigNum (strict)"(reference=w854) -> (error out=w853:errorcluster, "Value"=w852:sgl)  [unwired: 1 in, 1 out]
            n605 = property class="DigNum (strict)"(reference=w851, error in=w853, "Value"=w852) -> ()  [unwired: 2 out]
          }
          event "Bt_Ini_Exten": Value Change {
            n606 = event-data() -> ()  [unwired: 1 in, 6 out]
            n607 = Index Array(array=w857, index=8) -> (element=w855:string)
            n608 = call "Display Message to User5"("Message"=w855) -> ("OK"=w858:bool)  [unwired: 9 in, 1 out]
            n609 = case shown="True" w858 {
              tunnel: w859 -> [_ w862]
              frame False {
              }
              frame True {
                n610 = flat-sequence {
                  tunnel: w862 -> [w865]
                  tunnel: [w863] -> w860
                  tunnel: [w866] -> w861
                  tunnel: w860 -> [w866]
                  tunnel: w861 -> [w869]
                  frame #0 {
                    n611 = property class="Bool (strict)"(reference=w865, "Value"=TRUE) -> (reference out=w863:refnum<vi>)  [unwired: 1 in, 1 out]
                  }
                  frame #1 {
                    n612 = Wait Until Next ms Multiple(millisecond multiple=u32 200) -> ()  [unwired: 1 out]
                  }
                  frame #2 {
                    n613 = property class="Bool (strict)"(reference=w869, "Value"=FALSE) -> ()  [unwired: 1 in, 2 out]
                  }
                }
              }
            }
          }
          event "BtTaraF": Value Change {
            n614 = event-data() -> ()  [unwired: 1 in, 6 out]
            n615 = property class="DigNum (strict)"(reference=w872) -> ("Value"=w870:sgl)  [unwired: 1 in, 2 out]
            n616 = property class="DigNum (strict)"(reference=w871, "Value"=w870) -> ()  [unwired: 1 in, 2 out]
          }
          event "PrecargaOn": Value Change {
            n617 = event-data() -> ("NewVal"=w877:bool)  [unwired: 1 in, 5 out]
            n618 = case shown="True" w877 {
              tunnel: w876 -> [_ w881]
              tunnel: w875 -> [_ w879]
              tunnel: w874 -> [_ _]
              tunnel: w873 -> [_ _]
              frame False {
              }
              frame True {
                n619 = property class="DigNum (strict)"(reference=w881) -> (error out=w880:errorcluster, "Value"=w878:sgl)  [unwired: 1 in, 1 out]
                n620 = property class="DigNum (strict)"(reference=w879, error in=w880, "Value"=w878) -> ()  [unwired: 2 out]
              }
            }
          }
        }
        n621 = property on="Stop" class="Bool (strict)"() -> ("Value"=w540:bool)  [unwired: 2 in, 2 out]
      }
      n622 = call <vilib>:"DAQmx Stop Task.vi"("task/channels in"=w253, "error in"=w254) -> ("task out"=w256:refnum<k21>, "error out"=w255:errorcluster)  [unwired: 12 in]
      n623 = call <vilib>:"DAQmx Stop Task.vi"("task/channels in"=w261, "error in"=w260) -> ("task out"=w263:refnum<k21>, "error out"=w262:errorcluster)  [unwired: 12 in]
      n624 = call <vilib>:"DAQmx Clear Task.vi"("task in"=w256, "error in"=w255) -> ()  [unwired: 13 in, 1 out]
      n625 = call <vilib>:"DAQmx Clear Task.vi"("task in"=w263, "error in"=w262) -> ()  [unwired: 13 in, 1 out]
      n626 = control-ref of="Pujar"() -> (w234:refnum<vi>)
      n627 = control-ref of="Salir"() -> (w268:refnum<vi>)
      n628 = control-ref of="Velocidad Ensayo"() -> (w219:refnum<vi>)
      n629 = control-ref of="Velocidad Retorno"() -> (w218:refnum<vi>)
      n630 = control-ref of="VelocitatMàxima"() -> (w238:refnum<vi>)
      n631 = control-ref of="Mante_a_Vel_0"() -> (w211:refnum<vi>)
      n632 = control-ref of="Baixar"() -> (w233:refnum<vi>)
      n633 = control-ref of="MotorBipolar"() -> (w232:refnum<vi>)
      n634 = control-ref of="start"() -> (w235:refnum<vi>)
      n635 = call "SortidaAnalogicaUSB.vi"("VelocitatAssaig"=w219, "Mante_a_vel_0"=w211, "MotorBipolar"=w232, "stop"=w268, "Pujar"=w234, "Baixar"=w233, "VelocitatRetorn"=w218, "VelocitatMaxima"=w238, "AssaigActiu"=w235) -> ()  [unwired: 7 in]
      n636 = Unregister For Events(event registration refnum=w243) -> ()  [unwired: 1 in, 1 out]
      n637 = Current VI's Menubar() -> (w293:refnum<k9>)
      n638 = Delete Menu Items(9:w293) -> (3:w292:refnum<k9>)  [unwired: 3 in, 1 out]
      n639 = Insert Menu Items(8:string[] ["Calibra", "About"] ("item names"), 9:w292) -> (3:w240:refnum<k9>)  [unwired: 4 in, 2 out]
      n640 = while {
        tunnel: w240 -> [w435]
        stop <- w434 stop-if-true
        n641 = Get Menu Selection(0:w435, 1:200 ("ms timeout (200)")) -> (6:w436:string)  [unwired: 2 in, 4 out]
        n642 = case shown="\"Calibra\"" w436 {
          frame "About" {
            n643 = call "About.vi"() -> ()  [unwired: 1 in]
          }
          frame "Calibra" {
            n644 = control-ref of="Password"() -> (w440:refnum<vi>)
            n645 = property class="Str"(reference=w440) -> ("Value"=w439:string)  [unwired: 1 in, 2 out]
            n646 = call "Password.vi"() -> ("Password"=w441:string)  [unwired: 17 in, 2 out]
            n647 = Equal?(x=w439, y=w441) -> (x = y?=w438:bool)
            n648 = case shown="True" w438 {
              frame False {
              }
              frame True {
                n649 = call "Calibratge.vi"() -> ("OK ?"=w442:bool)  [unwired: 10 in]
                n650 = case shown="True" w442 {
                  frame False {
                  }
                  frame True {
                    n651 = control-ref of="Valor de control sobrecarga"() -> (w452:refnum<vi>)
                    n652 = call "ReadCal.vi"() -> ("SobrecargaC2"=w450:dbl, "BotoPresetExten"=w443:bool, "ResoExten"=w458:i8, "TextExtensometre"=w471:string, "TextDeformacio"=w470:string, "SegonCaptador"=w483:string, "MotorBipolar"=w446:bool, "UnitatsC2"=w494:string, "UnitatsC1"=w496:string, "PrimerCaptador"=w484:string, "ViuMotor"=w444:bool, "ExtenPoten"=w448:bool, "SobrecargaC1"=w451:dbl, "Password"=w509:string, "Pendents"=w464:dbl[], "VelocitatMàxima"=w456:dbl)  [unwired: 2 in, 10 out]
                    n653 = property on="ResoExten" class="Ring (strict)"("Value"=w458) -> ()  [unwired: 2 in, 2 out]
                    n654 = control-ref of="ValorSobrecargaC1"() -> (w455:refnum<vi>)
                    n655 = control-ref of="ValorSobrecargaC2"() -> (w454:refnum<vi>)
                    n656 = Decimal String To Number(string=w483) -> (number=w491:i32)  [unwired: 2 in, 1 out]
                    n657 = property on="Bt_Ini_Exten" class="Bool (strict)"("Visible"=w443) -> ()  [unwired: 2 in, 2 out]
                    n658 = property class="DigNum (strict)"(reference=w454, "Value"=w450) -> ()  [unwired: 1 in, 2 out]
                    n659 = Decimal String To Number(string=w484) -> (number=w492:i32)  [unwired: 2 in, 1 out]
                    n660 = control-ref of="ViuMotor"() -> (w445:refnum<vi>)
                    n661 = control-ref of="MotorBipolar"() -> (w447:refnum<vi>)
                    n662 = property on="Células" class="Ring (strict)"() -> ("StringsAndValues[]"=w490:T4)  [unwired: 2 in, 2 out]
                    n663 = property class="DigNum (strict)"(reference=w455, "Value"=w451) -> ()  [unwired: 1 in, 2 out]
                    n664 = control-ref of="ExtenPoten"() -> (w449:refnum<vi>)
                    n665 = property class="Bool (strict)"(reference=w449, "Value"=w448) -> ()  [unwired: 1 in, 2 out]
                    n666 = property class="Bool (strict)"(reference=w445, "Value"=w444) -> ()  [unwired: 1 in, 2 out]
                    n667 = property class="Bool (strict)"(reference=w447, "Value"=w446) -> ()  [unwired: 1 in, 2 out]
                    n668 = property on="CaptadorF" class="Ring (strict)"() -> ("Value"=w453:u16)  [unwired: 2 in, 2 out]
                    n669 = case shown="1" w453 {
                      tunnel: w452 -> [w511 w513]
                      tunnel: w451 -> [w510 _]
                      tunnel: w450 -> [_ w512]
                      frame 0, Default {
                        n670 = property class="DigNum (strict)"(reference=w511, "Value"=w510) -> ()  [unwired: 1 in, 2 out]
                      }
                      frame 1 {
                        n671 = property class="DigNum (strict)"(reference=w513, "Value"=w512) -> ()  [unwired: 1 in, 2 out]
                      }
                    }
                    n672 = control-ref of="ArraiUnitats"() -> (w495:refnum<vi>)
                    n673 = Index Array(array=w490, index=w492) -> (element=w482:cluster{"String":string, "Value":u8})
                    n674 = Index Array(array=w490, index=w491) -> (element=w488:cluster{"String":string, "Value":u8})
                    n675 = control-ref of="Pendents"() -> (w507:refnum<vi>)
                    n676 = Unbundle(w482) -> ("Value"=w481:u8)  [unwired: 1 out]
                    n677 = control-ref of="VelocitatMàxima"() -> (w457:refnum<vi>)
                    n678 = property class="DigNum (strict)"(reference=w457, "Value"=w456) -> ()  [unwired: 1 in, 2 out]
                    n679 = call "UnitatsStringsValors.vi"("UnitatsC1"=w496, "Arr Refnum"=w495) -> ("Array 2"=w486:cluster{"String":string, "Value":u16}[])  [unwired: 1 out]
                    n680 = call "UnitatsStringsValors.vi"("UnitatsC1"=w494, "Arr Refnum"=w495) -> ("Array 2"=w493:cluster{"String":string, "Value":u16}[])  [unwired: 1 out]
                    n681 = property class="Arr (strict)"(reference=w507, "Value"=w464) -> ()  [unwired: 1 in, 2 out]
                    n682 = Index Array(array=w464, index=3) -> (element=w468:dbl)
                    n683 = Unbundle(w488) -> ("Value"=w487:u8)  [unwired: 1 out]
                    n684 = property on="Password" class="Str"("Value"=w509) -> ()  [unwired: 2 in, 2 out]
                    n685 = property on="Celula_0" class="DigNum (strict)"("Value"=w481) -> ()  [unwired: 2 in, 2 out]
                    n686 = property on="UnidadesF_C2" class="Ring (strict)"("StringsAndValues[]"=w493) -> ()  [unwired: 2 in, 2 out]
                    n687 = Equal To 0?(x=w468) -> (x = 0?=w472:bool)
                    n688 = case shown="0, Default" w487 {
                      tunnel: w482 -> [w523 w524]
                      tunnel: w488 -> [w522 _]
                      tunnel: [w521 w525] -> w489
                      frame 0, Default {
                        n689 = Build Array(w523, w522) -> (w521:cluster{"String":string, "Value":u8}[])
                      }
                      frame 17 {
                        n690 = Build Array(w524) -> (w525:cluster{"String":string, "Value":u8}[])
                      }
                    }
                    n691 = case shown="False" w472 {
                      tunnel: w471 -> [w516 _]
                      tunnel: w470 -> [w517 w520]
                      tunnel: [w515 w519] -> w467
                      tunnel: [TRUE ("Extensometre") FALSE ("Extensometre")] -> w461
                      frame False {
                        n692 = Build Array(w517, w516) -> (w515:string[])
                      }
                      frame True {
                        n693 = Build Array(w520) -> (w519:string[])
                      }
                    }
                    n694 = property on="UnidadesF_C1" class="Ring (strict)"("StringsAndValues[]"=w486) -> ("Value"=w485:u16)  [unwired: 2 in, 2 out]
                    n695 = Index Array(array=w464, index=2) -> (element=w500:dbl)
                    n696 = Index Array(array=w464, index=0) -> (element=w501:dbl)
                    n697 = Index Array(array=w464, index=1) -> (element=w475:dbl)
                    n698 = Index Array(array=w464, index=3) -> (element=w474:dbl)
                    n699 = control-ref of="ConversioUnitatsD"() -> (w480:refnum<vi>)
                    n700 = Build Array(w501, w500) -> (w498:dbl[])
                    n701 = control-ref of="Calibratge"() -> (w499:refnum<vi>)
                    n702 = Build Array(w475, w474) -> (w473:dbl[])
                    n703 = control-ref of="ConversioUnitatsF"() -> (w508:refnum<vi>)
                    n704 = property on="Extensometre" class="Bool (strict)"("Value"=w461) -> ()  [unwired: 2 in, 2 out]
                    n705 = control-ref of="Calibratge D"() -> (w478:refnum<vi>)
                    n706 = property class="Arr (strict)"(reference=w480) -> ("Value"=w465:dbl[])  [unwired: 1 in, 2 out]
                    n707 = property class="Arr (strict)"(reference=w499, "Value"=w498) -> ()  [unwired: 1 in, 2 out]
                    n708 = property on="UnidadesF" class="Ring (strict)"("StringsAndValues[]"=w486, "Value"=w485) -> ()  [unwired: 2 in, 2 out]
                    n709 = property class="Arr (strict)"(reference=w478, "Value"=w473) -> ()  [unwired: 1 in, 2 out]
                    n710 = property class="Arr (strict)"(reference=w508) -> ("Value"=w506:dbl[])  [unwired: 1 in, 2 out]
                    n711 = Index Array(array=w464, index=0) -> (element=w497:dbl)
                    n712 = property on="CaptadorD" class="Ring (strict)"("Strings []"=w467, "Value"=0 ("index")) -> ()  [unwired: 2 in, 2 out]
                    n713 = Index Array(array=w464, index=1) -> (element=w463:dbl)
                    n714 = property on="CaptadorF" class="Ring (strict)"("StringsAndValues[]"=w489, "Value"=w481) -> ()  [unwired: 2 in, 2 out]
                    n715 = Multiply(x=w506, y=w497) -> (x*y=w504:dbl[])
                    n716 = control-ref of="FactorsUnitatsPendents_F"() -> (w505:refnum<vi>)
                    n717 = Multiply(x=w465, y=w463) -> (x*y=w462:dbl[])
                    n718 = control-ref of="FactorsUnitatsPendents_D"() -> (w479:refnum<vi>)
                    n719 = property class="Arr (strict)"(reference=w505, "Value"=w504) -> ()  [unwired: 1 in, 2 out]
                    n720 = property class="Arr (strict)"(reference=w479, "Value"=w462) -> ()  [unwired: 1 in, 2 out]
                  }
                }
              }
            }
          }
          frame Default {
          }
        }
        n721 = property on="Stop" class="Bool (strict)"() -> ("Value"=w434:bool)  [unwired: 2 in, 2 out]
      }
    }
    frame #5 {
      n722 = property on="rings" class="Arr (strict)"() -> ("Value"=w1191:refnum<vi>[])  [unwired: 2 in, 2 out]
      n723 = call "GuardaValorsPantalla.vi"("Rings"=w1191) -> ()  [unwired: 9 in, 1 out]
    }
    frame #6 {
      n724 = Quit LabVIEW(quit? (T)=TRUE) -> ()
    }
  }
